vi "运维调试_总磷总氮.vi"() -> ()   [LabVIEW 2016, in "斯坦道总磷.lvlib"]
uses:
  <vilib>/Utility/miscctls.llb/LVStringsAndValuesArrayTypeDef_U16.ctl
  <vilib>/Utility/miscctls.llb/LVPointTypeDef.ctl
  <vilib>/Plasmionique/MB Master/MB_Master/MB_Master.lvclass
  <vilib>/Utility/config.llb/NI_LVConfig.lvlib
  <vilib>/ptbypt/NI_PtbyPt.lvlib
panel:
  in  "测试量程配置":T1
  in  "启动参数设置":bool
  out "固件版本号":string
  in  "定时设置":cluster{"启动":bool, "控制命令":T2, "测量参数":T3}(xcontrol)
  out "模块版本号":string
  out "温度2":sgl
  out "温度1":sgl
  out "ADC":sgl
  out "F3":sgl format="%#.6f"
  out "F2":sgl format="%#.6f"
  out "F1":sgl format="%#.6f"
  out "F0":sgl format="%#.6f"
  out "运行状态":T4 {"数据时间:" format="%<%y/%m/%d %H:%M:%S>T"; "仪器时间:" format="%<%y/%m/%d %H:%M:%S>T"}
  in  "单选按钮":enum32{"COD", "NH3N", "TN", "TP"}(radio)=enum."TN"
  in  "仪器参数":bool
  out "二级权限":bool
  out "一级权限":bool
  out "输入密码":u32
  out "布尔":bool
  in  "流程固件":bool
  in  "量程参数读取":T5
  in  "模块启用":bool
  in  "串口设置":bool
  in  "公式一键写入":bool
  in  "流程路径":path=path "data/流程.xml"
  in  "曲线模型":cluster{"X^2":dbl, "X":dbl, "B":dbl, "r^2":dbl}(xcontrol)
  out "字符串 2":string
  in  "质控参数设置":bool
  in  "数组":string[](array[string])
  in  "量程切换阈值写入":bool
  in  "量程切换阈值读取":bool
  in  "参数下拉列表":enum16{"COD", "氨氮", "总氮", "总磷"}(ring)
  in  "量程下拉列表":enum16{"低量程", "高量程"}(ring)
  in  "测量模式下拉列表":enum16{"水样测量", "零点核查", "跨度核查", "标样核查", "加标回收"}(ring)
  in  "公式":cluster{"X^2":dbl, "X":dbl, "b":dbl}
  in  "写公式":bool
  in  "读公式":bool
  in  "返回":bool
  in  "参数设置":bool
  out "集成报警信息":string
  in  "停止":bool
  in  "手动启动":bool
  in  "单步测试":bool
  out "多列列表框":i32(listbox)
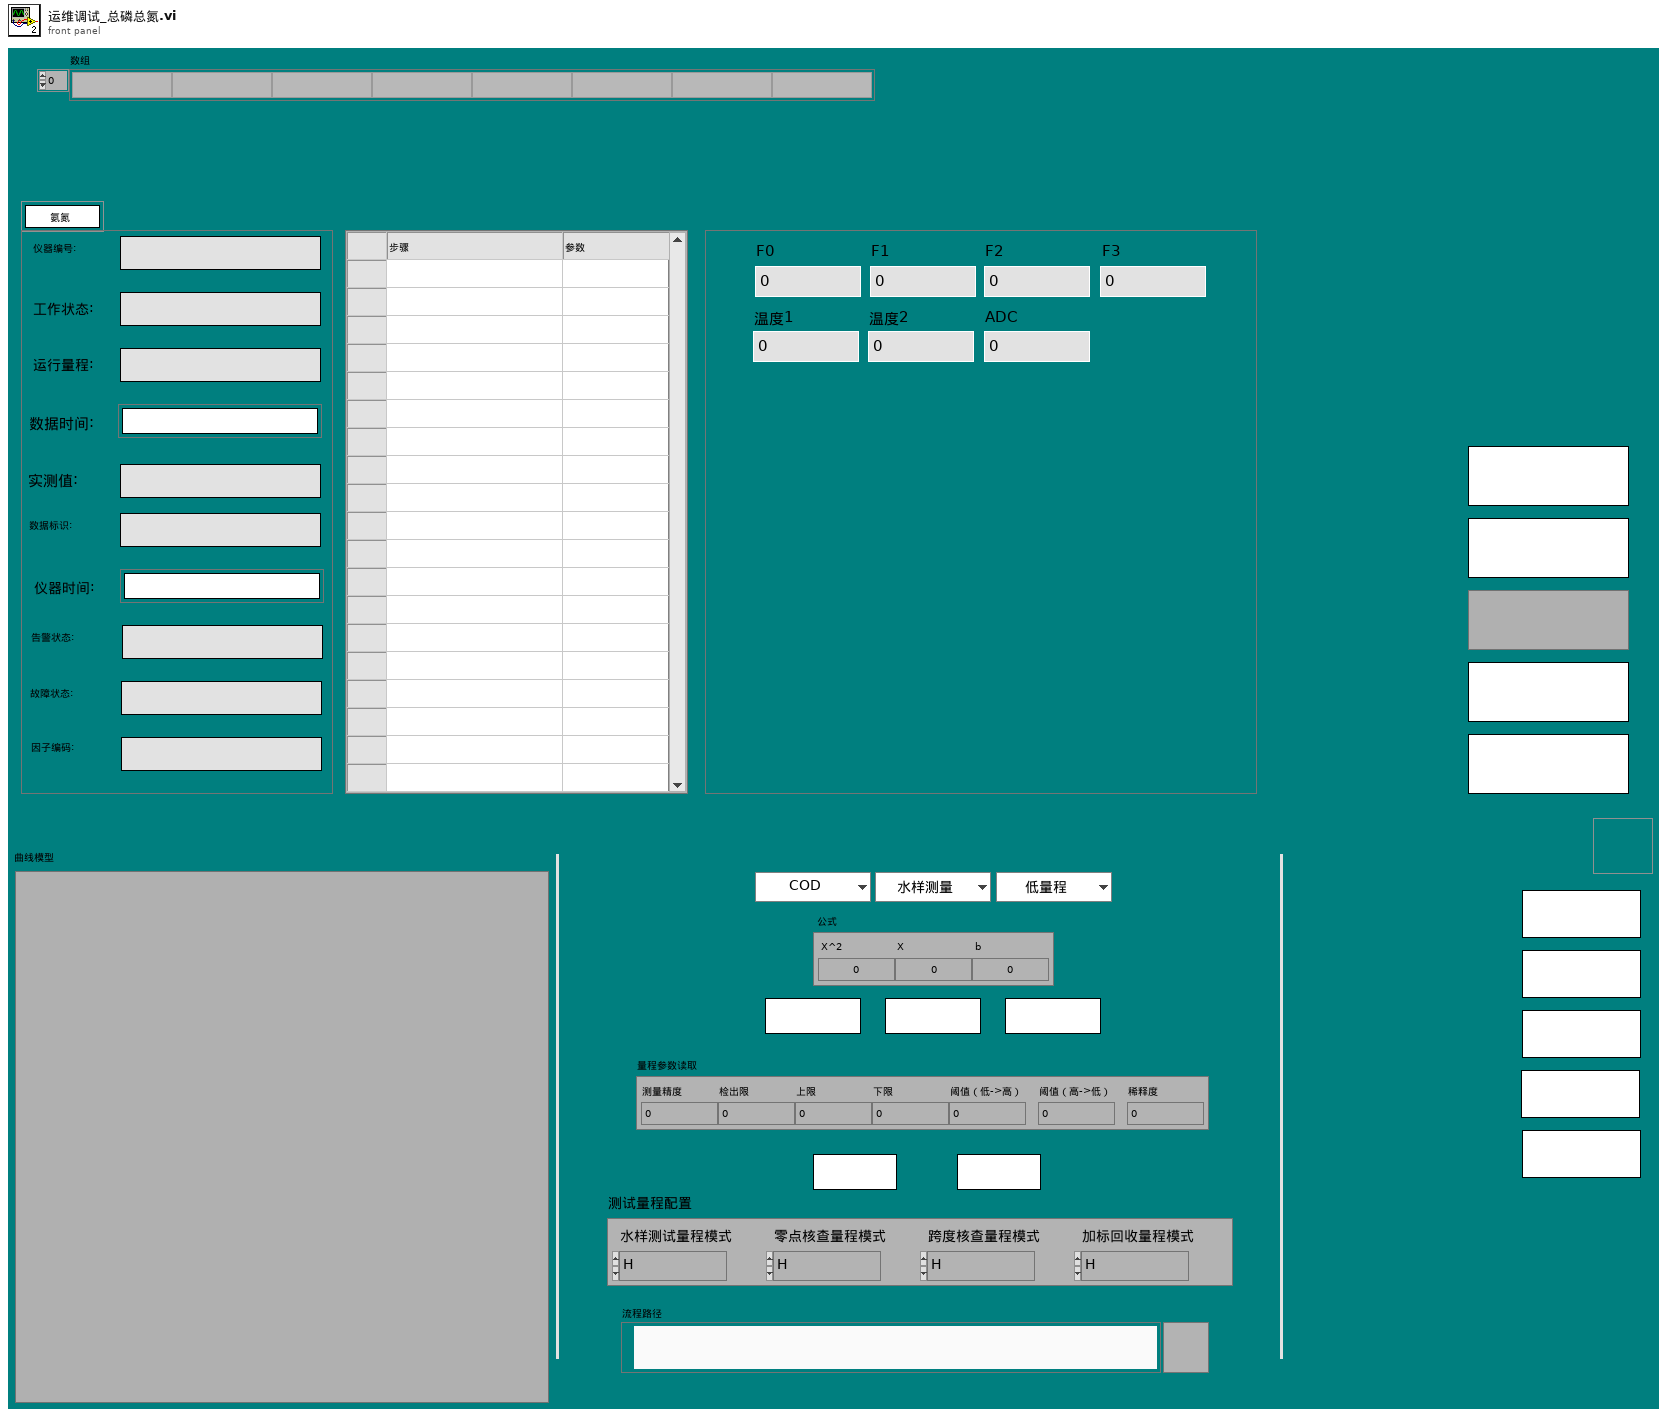
[diagram p1: front panel]
types:
  T1 = cluster{"水样测试量程模式":enum16{"H", "L", "AUTO"}, "空白核查量程模式":enum16{"H", "L", "AUTO"}, "跨度核查量程模式":enum16{"H", "L", "AUTO"}, "跨度核查量程模式 2":enum16{"H", "L", "AUTO"}}
  T2 = typedef "定时设置.xctl/国标控制命令.ctl" = enum16{"启动测量", "标样核查", "零点核查", "跨度核查", "空白测试", "平行样测试", "加标回收", "空白校准", "标样校准", "初始化（清洗）", "停止测试", "仪器重启", "校时", "模式设置", "测量间隔设置"}
  T3 = typedef "定时设置.xctl/测量参数.ctl" = u16
  T4 = cluster{"仪器编号:":string, "工作状态:":string, "运行量程: ":string, "数据时间:":timestamp, "实测值:":string, "数据标识: ":string, "仪器时间:":timestamp, "告警状态: ":string, "故障状态:  ":string, "因子编码:":string}
  T5 = cluster{"测量精度":dbl, "检出限":dbl, "上限":dbl, "下限":dbl, "阈值（低->高）":dbl, "阈值（高->低）":dbl, "稀释度":dbl}
  T6 = cluster{"时间源选择":enum16{"系统时间源", "仪器时间源"}, "外部时间源":timestamp}
  T7 = cluster{"系统时间":timestamp, "工作状态":enum16{"空闲", "水样测试", "标样核查", "零点核查", "跨度核查", "空白测试", "平行样测试", "加标回收", "空白校准", "标样校准", "初始化（清洗）"}, "测量模式":enum16{"待机", "连续模式", "周期模式", "定点模式", "受控模式", "手动模式"}, "告警代码":u16, "故障代码":u16, "日志代码":u16, "软件版本":u16, "F0":sgl, "F1":sgl, "F2":sgl, "F3":sgl, "T":sgl, "H":sgl, "id":u16, "flowid":u16, "量程":u16, "总磷控温温度1":sgl, "营养盐控温温度2":sgl, "ADC":sgl}
  T8 = enum32{"Bad", "Idle", "Run top level", "Running"}
  T9 = enum16{"空闲", "水样测试", "标样核查", "零点核查", "跨度核查", "空白测试", "平行样测试", "加标回收", "空白校准", "标样校准", "初始化（清洗）"}
  T10 = cluster{"水样测试量程模式":enum16{"H", "L", "AUTO"}, "空白核查量程模式":enum16{"H", "L", "AUTO"}, "跨度核查量程模式":enum16{"H", "L", "AUTO"}, "加标回收量程模式":enum16{"H", "L", "AUTO"}}
  T11 = typedef "LVStringsAndValuesArrayTypeDef_U16.ctl" = cluster{"String":string, "Value":u16}[]
  T12 = cluster{"COD":bool, "氨氮":bool, "总氮":bool, "总磷":bool}
  T13 = typedef "NI_LVConfig.lvlib/Config Data RefNum.ctl" = refnum<k1>
  T14 = cluster{"Major":u16, "Minor":u16, "Fix":u16, "Build":u16}
  T15 = cluster{i32, "测量模式下拉列表":enum16{"水样测量", "零点核查", "跨度核查", "标样核查", "加标回收"}, "量程下拉列表":enum16{"低量程", "高量程"}}
  T16 = typedef "LVPointTypeDef.ctl" = cluster{"Horizontal":i16, "Vertical":i16}
  T17 = cluster{"因子编码":u32, "单位":u16, "标样参考值":sgl, "水样数据时间":timestamp, "水样实测值":sgl, "水样数据标识":string, "标样数据时间":timestamp, "标样实测值":sgl, "标样数据标识":string, "空白数据时间":timestamp, "空白实测值":sgl, "空白数据标识":string, "零点核查数据时间":timestamp, "零点核查实测值":sgl, "零点核查数据标识":string, "跨度核查数据时间":timestamp, "跨度核查实测值":sgl, "跨度核查数据标识":string, "加标回收数据时间":timestamp, "加标回收实测值":sgl, "加标回收数据标识":string, "平行样数据时间":timestamp, "平行样实测值":sgl, "平行样数据标识":string, "F0":sgl, "F1":sgl, "F2":sgl, "F3":sgl, "F4":sgl, "F5":sgl, "F6":sgl, "F7":sgl, "温度":sgl, "湿度":sgl, "X值":sgl, "fidrange":u16}
  T18 = cluster{"时间标识":timestamp, "设备":string, "日志信息":string, "备注":string}
  T19 = cluster{"参数":string, "报警内容":string, "报警分析":string}
  T20 = cluster{"启动模式":enum16{"跨度核查", "水样测量", "空白核查", "标样核查", "加标回收"}, "启动参数":u16, "量程":enum16{"低量程", "高量程"}}
  T21 = cluster{"时间标识":timestamp, "设备":string, "日志信息":string, "流程参数":string}
  T22 = typedef "LVRowAndColumnUnsignedTypeDef.ctl" = cluster{"Row":u32, "Column":u32}
  T23 = cluster{"站号":u16, "量程切换":enum32{"H", "L", "AUTO"}, "控制命令":enum16{"启动测量", "标样核查", "零点核查", "跨度核查", "空白测试", "平行样测试", "加标回收", "空白校准", "标样校准", "初始化（清洗）", "停止测试", "仪器重启", "校时", "模式设置", "测量间隔设置"}, "模式设置":enum16{"待机", "连续模式", "周期模式", "定点模式", "受控模式", "手动模式"}, "测量间隔":u16}
  T24 = cluster{"参数下拉列表":enum16{"COD", "氨氮", "总氮", "总磷"}, "测量模式下拉列表":enum16{"水样测量", "零点核查", "跨度核查", "标样核查", "加标回收"}, "量程下拉列表":enum16{"低量程", "高量程"}}
  T25 = cluster{"被复制模型":cluster{"参数":u8, "测量模式":u8, "量程":u8}, "被覆盖模型":cluster{"参数":u8, "测量模式":u8, "量程":u8}[]}
  T26 = cluster{"总磷跨度值":dbl, "总磷零点标准液浓度":dbl, "总磷跨度标准液浓度":dbl, "总磷标准液标准浓度":dbl, "总氮跨度值":dbl, "总氮零点标准液浓度":dbl, "总氮跨度标准液浓度":dbl, "总氮标准液标准浓度":dbl, "COD跨度值":dbl, "COD零点标准液浓度":dbl, "COD跨度标准液浓度":dbl, "COD标准液标准浓度":dbl, "氨氮跨度值":dbl, "氨氮零点标准液浓度":dbl, "氨氮跨度标准液浓度":dbl, "氨氮标准液标准浓度":dbl}
  T27 = cluster{"测量量程":dbl, "测量精度":dbl, "测量间隔":dbl, "消解温度":dbl, "消解时长":dbl, "空白校准时间":timestamp, "曲线截距":dbl, "曲线斜率":dbl, "测量检出限":dbl, "测量信号值":dbl, "线性相关系数":dbl, "二次多项式系数":dbl, "标样校准时间":timestamp, "稀释倍数":dbl, "三项式系数":dbl, "空白标定系数":dbl, "量程系数":dbl, "F0/ORPA":dbl, "F1/ORPB":dbl, "F2/ORPK":dbl, "F3":dbl, "F4":dbl, "F5":dbl, "F6":dbl, "F7":dbl, "X0/滴定数":dbl, "量程":dbl}
  T28 = cluster{"COD仪器参数":cluster{"测量量程":dbl, "测量精度":dbl, "测量间隔":dbl, "消解温度":dbl, "消解时长":dbl, "空白校准时间":timestamp, "曲线截距":dbl, "曲线斜率":dbl, "测量检出限":dbl, "测量信号值":dbl, "线性相关系数":dbl, "二次多项式系数":dbl, "标样校准时间":timestamp, "稀释倍数":dbl, "三项式系数":dbl, "空白标定系数":dbl, "量程系数":dbl, "F0/ORPA":dbl, "F1/ORPB":dbl, "F2/ORPK":dbl, "F3":dbl, "F4":dbl, "F5":dbl, "F6":dbl, "F7":dbl, "X0/滴定数":dbl, "量程":dbl}, "氨氮仪器参数":cluster{"测量量程":dbl, "测量精度":dbl, "测量间隔":dbl, "消解温度":dbl, "消解时长":dbl, "空白校准时间":timestamp, "曲线截距":dbl, "曲线斜率":dbl, "测量检出限":dbl, "测量信号值":dbl, "线性相关系数":dbl, "二次多项式系数":dbl, "标样校准时间":timestamp, "稀释倍数":dbl, "三项式系数":dbl, "空白标定系数":dbl, "量程系数":dbl, "F0/ORPA":dbl, "F1/ORPB":dbl, "F2/ORPK":dbl, "F3":dbl, "F4":dbl, "F5":dbl, "F6":dbl, "F7":dbl, "X0/滴定数":dbl, "量程":dbl}, "总氮仪器参数":cluster{"测量量程":dbl, "测量精度":dbl, "测量间隔":dbl, "消解温度":dbl, "消解时长":dbl, "空白校准时间":timestamp, "曲线截距":dbl, "曲线斜率":dbl, "测量检出限":dbl, "测量信号值":dbl, "线性相关系数":dbl, "二次多项式系数":dbl, "标样校准时间":timestamp, "稀释倍数":dbl, "三项式系数":dbl, "空白标定系数":dbl, "量程系数":dbl, "F0/ORPA":dbl, "F1/ORPB":dbl, "F2/ORPK":dbl, "F3":dbl, "F4":dbl, "F5":dbl, "F6":dbl, "F7":dbl, "X0/滴定数":dbl, "量程":dbl}, "总磷仪器参数":cluster{"测量量程":dbl, "测量精度":dbl, "测量间隔":dbl, "消解温度":dbl, "消解时长":dbl, "空白校准时间":timestamp, "曲线截距":dbl, "曲线斜率":dbl, "测量检出限":dbl, "测量信号值":dbl, "线性相关系数":dbl, "二次多项式系数":dbl, "标样校准时间":timestamp, "稀释倍数":dbl, "三项式系数":dbl, "空白标定系数":dbl, "量程系数":dbl, "F0/ORPA":dbl, "F1/ORPB":dbl, "F2/ORPK":dbl, "F3":dbl, "F4":dbl, "F5":dbl, "F6":dbl, "F7":dbl, "X0/滴定数":dbl, "量程":dbl}}
  T29 = cluster{"测量精度":u16, "检出限":dbl, "上限":dbl, "下限":dbl, "阈值（低->高）":dbl, "阈值（高->低）":dbl, "稀释度":dbl}
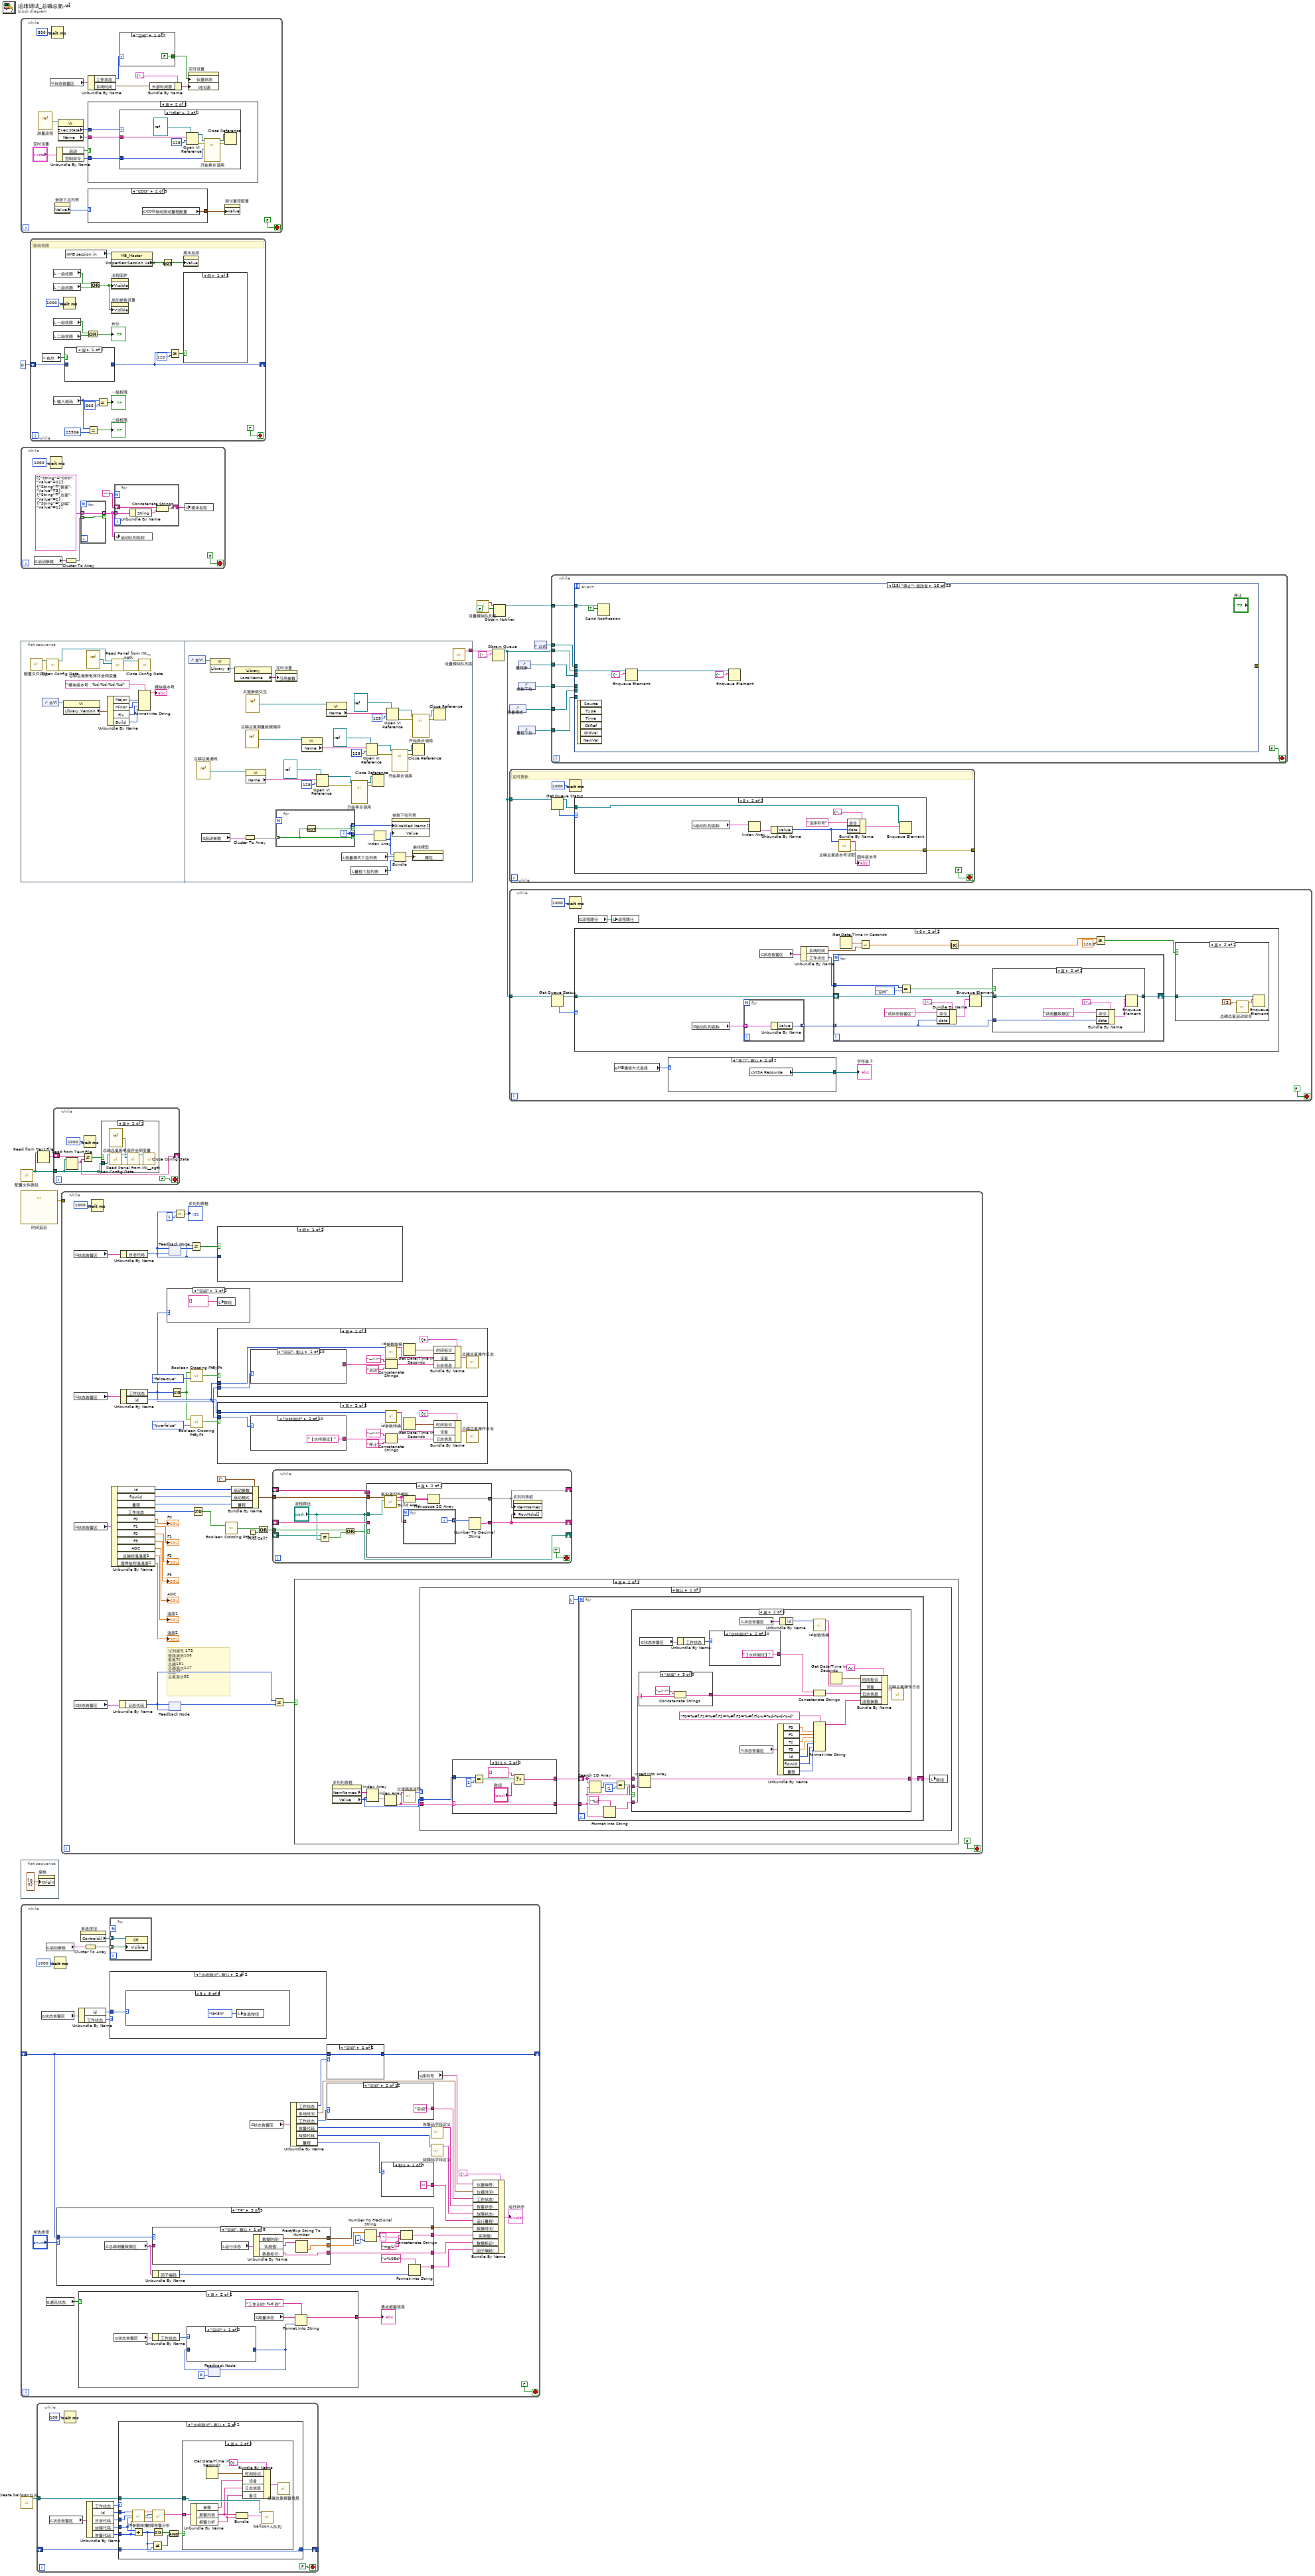
[diagram p0: block diagram]
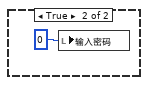
[diagram p5: hidden frame]
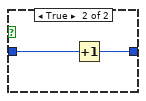
[diagram p6: hidden frame]
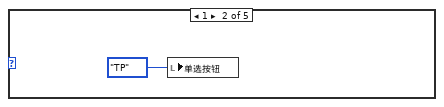
[diagram p11: hidden frame]
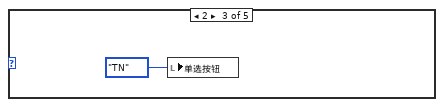
[diagram p12: hidden frame]
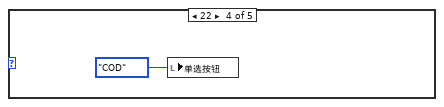
[diagram p13: hidden frame]
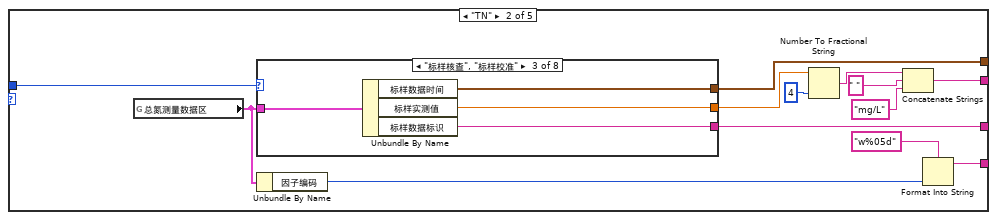
[diagram p15: hidden frame]
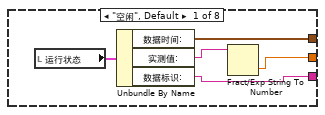
[diagram p16: hidden frame]
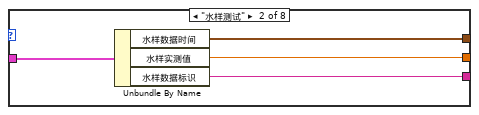
[diagram p17: hidden frame]
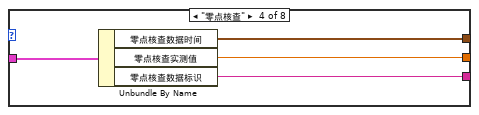
[diagram p18: hidden frame]
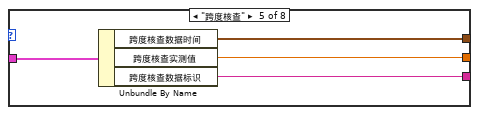
[diagram p19: hidden frame]
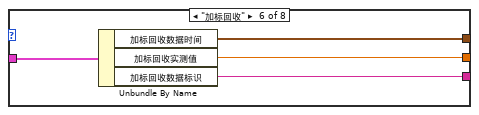
[diagram p20: hidden frame]
diagram:
  n1 = while {
    stop <- FALSE stop-if-true
    n2 = vi-ref "测量流程.vi"() -> (w30:refnum<vi>)
    n3 = global read "VAR总磷总氮全局变量.vi" "状态告警区"() -> (w27:T7)
    n4 = Wait (ms)(milliseconds to wait=u32 500 ("等待时间（毫秒）")) -> ()  [unwired: 1 out]
    n5 = property on="参数下拉列表" class="Enum (严格)"() -> ("Value"=w19:enum16{"COD", "氨氮", "总氮", "总磷"})  [unwired: 2 in, 2 out]
    n6 = Unbundle By Name("定时设置") -> ("启动"=w24:bool, "控制命令"=w23:T2)
    n7 = property class="VI"(reference=w30) -> ("Exec.State"=w29:T8, "Name"=w28:string)  [unwired: 1 in, 2 out]
    n8 = Unbundle By Name(w27) -> ("工作状态"=w26:T9, "系统时间"=w21:timestamp)
    n9 = case shown="真" w24 {
      tunnel: w28 -> [_ w41]
      tunnel: w23 -> [_ w40]
      tunnel: w29 -> [_ w39]
      frame False {
      }
      frame True {
        n10 = case shown="\"Idle\"" w39 {
          tunnel: w41 -> [_ w45]
          tunnel: w40 -> [_ w42]
          frame "Bad", Default {
          }
          frame "Idle" {
            n11 = Open VI Reference(type specifier VI Refnum (for type only)=refnum<vi> refnum, vi path=w45, options=128 ("选项")) -> (vi reference=w46:refnum<vi>, error out=w47:errorcluster)  [unwired: 3 in]
            n12 = call-by-ref "开始异步调用"(reference=w46, error in=w47, "控制命令"=w42) -> (reference out=w48:refnum<vi>, error out=w49:errorcluster)  [unwired: 11 in]
            n13 = Close Reference(reference=w48, error in (no error)=w49) -> ()  [unwired: 1 out]
          }
        }
      }
    }
    n14 = case shown="\"COD\"" w19 {
      tunnel: [_ w33 w34 w35 w36] -> w18
      frame Default {
      }
      frame "COD" {
        n15 = global read "总磷总氮断电保存全局变量.vi" "COD自动测试量程配置"() -> (w33:T10)
      }
      frame "氨氮" {
        n16 = global read "总磷总氮断电保存全局变量.vi" "氨氮自动测试量程配置"() -> (w34:T10)
      }
      frame "总氮" {
        n17 = global read "总磷总氮断电保存全局变量.vi" "总氮自动测试量程配置"() -> (w35:T10)
      }
      frame "总磷" {
        n18 = global read "总磷总氮断电保存全局变量.vi" "总磷自动测试量程配置"() -> (w36:T10)
      }
    }
    n19 = case shown="\"空闲\"" w26 {
      tunnel: [FALSE TRUE] -> w17
      frame "空闲" {
      }
      frame "水样测试", Default {
      }
    }
    n20 = Bundle By Name(cluster=T6 {"时间源选择"=enum."仪器时间源", "外部时间源"=timestamp(0 s since 1904-01-01)} ("时间源"), "外部时间源"=w21) -> (w20:T6)
    n21 = property on="定时设置" class="定时设置 (严格)"("仪器状态"=w17, "时间源"=w20) -> ()  [unwired: 2 in, 2 out]
    n22 = property on="测试量程配置" class="Clust (严格)"("Value"=w18) -> ()  [unwired: 2 in, 2 out]
  }
  n23 = while {
    stop <- FALSE stop-if-true
    n24 = global read "总磷总氮断电保存全局变量.vi" "启动参数"() -> (w55:T12)
    n25 = Wait (ms)(milliseconds to wait=u32 1000 ("等待时间（毫秒）")) -> ()  [unwired: 1 out]
    n26 = Cluster To Array(cluster=w55) -> (array=w54:bool[])
    n27 = for {
      tunnel: w54 -> [w63] mode=indexing
      tunnel: T11 [{"String"="COD", "Value"=22}, {"String"="氨氮", "Value"=3}, {"String"="总氮", "Value"=2}, {"String"="总磷", "Value"=1}] ("字符串与值[]") -> [w62] mode=indexing
      tunnel: [w62] -> w52 mode=indexing if=w63
    }
    n28 = for {
      tunnel: w52 -> [w61] mode=indexing
      shift-right: [w60] -> w50
      shift-left: "" -> [w58]
      n29 = Unbundle By Name(w61) -> ("String"=w59:string)
      n30 = Concatenate Strings(w58, w59) -> (w60:string)
    }
    n31 = global write "VAR总磷总氮全局变量.vi" "启动队列名称"(w52) -> ()
    n32 = global write "VAR总磷总氮全局变量.vi" "模块名称"(w50) -> ()
  }
  n33 = flat-sequence {
    tunnel: [w78] -> w6
    frame #0 {
      n34 = call "配置文件路径.vi"() -> ("appended path"=w72:path)  [unwired: 11 in]
      n35 = control-ref of="本VI"() -> (w71:refnum<vi>)
      n36 = call <vilib>:"Open Config Data.vi"("configuration file path"=w72) -> ("error out"=w76:errorcluster, "refnum"=w73:T13)  [unwired: 8 in, 1 out]
      n37 = property class="VI"(reference=w71) -> ("Library.Version"=w70:T14)  [unwired: 1 in, 2 out]
      n38 = vi-ref "总磷总氮断电保存全局变量.vi"() -> (w74:refnum<vi>)
      n39 = Unbundle By Name(w70) -> ("Major"=w68:u16, "Minor"=w67:u16, "Fix"=w66:u16, "Build"=w65:u16)
      n40 = call <userlib>:"Read Panel from INI__ogtk.vi"("error in (no error)"=w76, "VI ref"=w74, "refnum"=w73) -> ("error out"=w77:errorcluster, "refnum out"=w75:T13)  [unwired: 7 in]
      n41 = call <vilib>:"Close Config Data.vi"("error in (no error)"=w77, "refnum"=w75) -> ()  [unwired: 8 in, 2 out]
      n42 = Format Into String(format string="模块版本号：%d.%d.%d.%d" ("格式字符串"), w68, w67, w66, w65) -> (resulting string=→"模块版本号":string)  [unwired: 2 in, 1 out]
    }
    frame #1 {
      n43 = control-ref of="本VI"() -> (w80:refnum<vi>)
      n44 = vi-ref "总磷总氮通讯.vi"() -> (w98:refnum<vi>)
      n45 = global read "总磷总氮断电保存全局变量.vi" "启动参数"() -> (w86:T12)
      n46 = property class="VI"(reference=w80) -> ("Library"=w81:refnum<vi>)  [unwired: 1 in, 2 out]
      n47 = property class="Library"(reference=w81) -> ("LocalName"=w82:string)  [unwired: 1 in, 2 out]
      n48 = Cluster To Array(cluster=w86) -> (array=w87:bool[])
      n49 = vi-ref "总磷总氮测量数据储存.vi"() -> (w106:refnum<vi>)
      n50 = vi-ref "关键参数交互.vi"() -> (w97:refnum<vi>)
      n51 = property class="VI"(reference=w98) -> ("Name"=w99:string)  [unwired: 1 in, 2 out]
      n52 = property on="定时设置" class="定时设置 (严格)"("引用参数"=w82) -> ()  [unwired: 2 in, 2 out]
      n53 = for {
        tunnel: w87 -> [w114] mode=indexing
        tunnel: [w115] -> w89 mode=indexing if=w116
        tunnel: [w115] -> w88 mode=indexing if=w114
        i -> [w115]
        n54 = Not(x=w114) -> (.not. x?=w116:bool)
      }
      n55 = property class="VI"(reference=w106) -> ("Name"=w113:string)  [unwired: 1 in, 2 out]
      n56 = Open VI Reference(type specifier VI Refnum (for type only)=refnum<vi> refnum, vi path=w99, options=128 ("选项")) -> (vi reference=w101:refnum<vi>, error out=w103:errorcluster)  [unwired: 3 in]
      n57 = property class="VI"(reference=w97) -> ("Name"=w91:string)  [unwired: 1 in, 2 out]
      n58 = local read "测量模式下拉列表"() -> (w84:enum16{"水样测量", "零点核查", "跨度核查", "标样核查", "加标回收"})
      n59 = local read "量程下拉列表"() -> (w83:enum16{"低量程", "高量程"})
      n60 = call-by-ref "开始异步调用"(reference=w101, error in=w103) -> (reference out=w105:refnum<vi>, error out=w104:errorcluster)  [unwired: 12 in]
      n61 = Open VI Reference(type specifier VI Refnum (for type only)=refnum<vi> refnum, vi path=w113, options=128 ("选项")) -> (vi reference=w111:refnum<vi>, error out=w109:errorcluster)  [unwired: 3 in]
      n62 = Close Reference(reference=w105, error in (no error)=w104) -> ()  [unwired: 1 out]
      n63 = Index Array(array=w88) -> (element=w79:i32)  [unwired: 1 in]
      n64 = Open VI Reference(type specifier VI Refnum (for type only)=refnum<vi> refnum, vi path=w91, options=128 ("选项")) -> (vi reference=w93:refnum<vi>, error out=w94:errorcluster)  [unwired: 3 in]
      n65 = call-by-ref "开始异步调用"(reference=w111, error in=w109) -> (reference out=w107:refnum<vi>, error out=w108:errorcluster)  [unwired: 12 in]
      n66 = property on="参数下拉列表" class="Enum (严格)"("Disabled Items []"=w89, "Value"=w79) -> ()  [unwired: 2 in, 2 out]
      n67 = Bundle(w79, "测量模式下拉列表"=w84, "量程下拉列表"=w83) -> (w85:T15)  [unwired: 1 in]
      n68 = call-by-ref "开始异步调用"(reference=w93, error in=w94) -> (reference out=w96:refnum<vi>, error out=w95:errorcluster)  [unwired: 12 in]
      n69 = Close Reference(reference=w107, error in (no error)=w108) -> ()  [unwired: 1 out]
      n70 = property on="曲线模型" class="曲线模型 (严格)"("属性"=w85) -> ()  [unwired: 2 in, 2 out]
      n71 = Close Reference(reference=w96, error in (no error)=w95) -> ()  [unwired: 1 out]
      n72 = call "设置模块队列名.vi"() -> ("Msg"=w78:string)  [unwired: 5 in]
    }
  }
  n73 = call "配置文件路径.vi"() -> ("appended path"=w4:path)  [unwired: 11 in]
  n74 = call "时间延迟"() -> ("error out"=w11:errorcluster)  [unwired: 11 in]
  n75 = flat-sequence {
    frame #0 {
      n76 = property on="窗格" class="Pane"("Origin"=T16 {"Horizontal"=0, "Vertical"=0} ("原点")) -> ()  [unwired: 2 in, 2 out]
    }
  }
  n77 = while {
    shift-right: [w119] -> _
    shift-left: _ -> [w118]
    stop <- FALSE stop-if-true
    n78 = global read "VAR总磷总氮全局变量.vi" "状态告警区"() -> (w130:T7)
    n79 = global read "总磷总氮断电保存全局变量.vi" "启动参数"() -> (w122:T12)
    n80 = global read "VAR总磷总氮全局变量.vi" "通讯状态"() -> (w146:bool)
    n81 = Wait (ms)(milliseconds to wait=u32 1000 ("等待时间（毫秒）")) -> ()  [unwired: 1 out]
    n82 = case shown="\"TP\"" "单选按钮" {
      tunnel: w118 -> [_ w162 w208 w254 w300]
      tunnel: [_ w161 w207 w252 w298] -> w134
      tunnel: [_ w160 w210 w256 w302] -> w133
      tunnel: [_ w159 w205 w250 w296] -> w132
      tunnel: [_ w158 w209 w255 w301] -> w131
      frame Default {
      }
      frame "TN" {
        n83 = global read "VAR总磷总氮全局变量.vi" "总氮测量数据区"() -> (w163:T17)
        n84 = case shown="\"标样核查\", \"标样校准\"" w162 {
          tunnel: [w173 w179 w183 w187 w191 w195 w199 w203] -> w161
          tunnel: [w171 w178 w182 w186 w189 w194 w198 w202] -> w165
          tunnel: [w174 w177 w181 w185 w188 w193 w197 w201] -> w159
          tunnel: w163 -> [_ w176 w180 w184 w190 w192 w196 w200]
          frame "空闲", Default {
            n85 = local read "运行状态"() -> (w175:T4)
            n86 = Unbundle By Name(w175) -> ("数据时间:"=w173:timestamp, "实测值:"=w172:string, "数据标识:"=w174:string)
            n87 = Fract/Exp String To Number(string=w172) -> (number=w171:dbl)  [unwired: 3 in, 1 out]
          }
          frame "水样测试" {
            n88 = Unbundle By Name(w176) -> ("水样数据时间"=w179:timestamp, "水样实测值"=w178:sgl, "水样数据标识"=w177:string)
          }
          frame "标样核查", "标样校准" {
            n89 = Unbundle By Name(w180) -> ("标样数据时间"=w183:timestamp, "标样实测值"=w182:sgl, "标样数据标识"=w181:string)
          }
          frame "零点核查" {
            n90 = Unbundle By Name(w184) -> ("零点核查数据时间"=w187:timestamp, "零点核查实测值"=w186:sgl, "零点核查数据标识"=w185:string)
          }
          frame "跨度核查" {
            n91 = Unbundle By Name(w190) -> ("跨度核查数据时间"=w191:timestamp, "跨度核查实测值"=w189:sgl, "跨度核查数据标识"=w188:string)
          }
          frame "加标回收" {
            n92 = Unbundle By Name(w192) -> ("加标回收数据时间"=w195:timestamp, "加标回收实测值"=w194:sgl, "加标回收数据标识"=w193:string)
          }
          frame "空白测试", "空白校准" {
            n93 = Unbundle By Name(w196) -> ("空白数据时间"=w199:timestamp, "空白实测值"=w198:sgl, "空白数据标识"=w197:string)
          }
          frame "平行样测试" {
            n94 = Unbundle By Name(w200) -> ("平行样数据时间"=w203:timestamp, "平行样实测值"=w202:sgl, "平行样数据标识"=w201:string)
          }
        }
        n95 = Unbundle By Name(w163) -> ("因子编码"=w169:u32)
        n96 = Number To Fractional String(number=w165, precision (6)=i16 4 ("精度(6)")) -> (F-format string=w167:string)  [unwired: 2 in]
        n97 = Concatenate Strings(w167, " " ("字符串"), "mg/L" ("字符串")) -> (w160:string)
        n98 = Format Into String(format string="w%05d" ("格式字符串"), w169) -> (resulting string=w158:string)  [unwired: 2 in, 1 out]
      }
      frame "TP" {
        n99 = global read "VAR总磷总氮全局变量.vi" "总磷测量数据区"() -> (w204:T17)
        n100 = case shown="\"空闲\", 默认" w208 {
          tunnel: [w219 w225 w229 w233 w237 w241 w245 w249] -> w207
          tunnel: [w217 w224 w228 w232 w235 w240 w244 w248] -> w206
          tunnel: [w220 w223 w227 w231 w234 w239 w243 w247] -> w205
          tunnel: w204 -> [_ w222 w226 w230 w236 w238 w242 w246]
          frame "空闲", Default {
            n101 = local read "运行状态"() -> (w221:T4)
            n102 = Unbundle By Name(w221) -> ("数据时间:"=w219:timestamp, "实测值:"=w218:string, "数据标识:"=w220:string)
            n103 = Fract/Exp String To Number(string=w218) -> (number=w217:dbl)  [unwired: 3 in, 1 out]
          }
          frame "水样测试" {
            n104 = Unbundle By Name(w222) -> ("水样数据时间"=w225:timestamp, "水样实测值"=w224:sgl, "水样数据标识"=w223:string)
          }
          frame "标样核查" {
            n105 = Unbundle By Name(w226) -> ("标样数据时间"=w229:timestamp, "标样实测值"=w228:sgl, "标样数据标识"=w227:string)
          }
          frame "零点核查" {
            n106 = Unbundle By Name(w230) -> ("零点核查数据时间"=w233:timestamp, "零点核查实测值"=w232:sgl, "零点核查数据标识"=w231:string)
          }
          frame "跨度核查" {
            n107 = Unbundle By Name(w236) -> ("跨度核查数据时间"=w237:timestamp, "跨度核查实测值"=w235:sgl, "跨度核查数据标识"=w234:string)
          }
          frame "加标回收" {
            n108 = Unbundle By Name(w238) -> ("加标回收数据时间"=w241:timestamp, "加标回收实测值"=w240:sgl, "加标回收数据标识"=w239:string)
          }
          frame "空白测试" {
            n109 = Unbundle By Name(w242) -> ("空白数据时间"=w245:timestamp, "空白实测值"=w244:sgl, "空白数据标识"=w243:string)
          }
          frame "平行样测试" {
            n110 = Unbundle By Name(w246) -> ("平行样数据时间"=w249:timestamp, "平行样实测值"=w248:sgl, "平行样数据标识"=w247:string)
          }
        }
        n111 = Unbundle By Name(w204) -> ("因子编码"=w215:u32)
        n112 = Number To Fractional String(number=w206, precision (6)=i16 4 ("精度(6)")) -> (F-format string=w213:string)  [unwired: 2 in]
        n113 = Concatenate Strings(w213, " " ("字符串"), "mg/L" ("字符串")) -> (w210:string)
        n114 = Format Into String(format string="w%05d" ("格式字符串"), w215) -> (resulting string=w209:string)  [unwired: 2 in, 1 out]
      }
      frame "NH3N" {
        n115 = global read "VAR总磷总氮全局变量.vi" "氨氮测量数据区"() -> (w253:T17)
        n116 = case shown="\"空闲\", 默认" w254 {
          tunnel: [w265 w271 w275 w279 w283 w287 w291 w295] -> w252
          tunnel: [w263 w270 w274 w278 w281 w286 w290 w294] -> w251
          tunnel: [w266 w269 w273 w277 w280 w285 w289 w293] -> w250
          tunnel: w253 -> [_ w268 w272 w276 w282 w284 w288 w292]
          frame "空闲", Default {
            n117 = local read "运行状态"() -> (w267:T4)
            n118 = Unbundle By Name(w267) -> ("数据时间:"=w265:timestamp, "实测值:"=w264:string, "数据标识:"=w266:string)
            n119 = Fract/Exp String To Number(string=w264) -> (number=w263:dbl)  [unwired: 3 in, 1 out]
          }
          frame "水样测试" {
            n120 = Unbundle By Name(w268) -> ("水样数据时间"=w271:timestamp, "水样实测值"=w270:sgl, "水样数据标识"=w269:string)
          }
          frame "标样核查" {
            n121 = Unbundle By Name(w272) -> ("标样数据时间"=w275:timestamp, "标样实测值"=w274:sgl, "标样数据标识"=w273:string)
          }
          frame "零点核查" {
            n122 = Unbundle By Name(w276) -> ("零点核查数据时间"=w279:timestamp, "零点核查实测值"=w278:sgl, "零点核查数据标识"=w277:string)
          }
          frame "跨度核查" {
            n123 = Unbundle By Name(w282) -> ("跨度核查数据时间"=w283:timestamp, "跨度核查实测值"=w281:sgl, "跨度核查数据标识"=w280:string)
          }
          frame "加标回收" {
            n124 = Unbundle By Name(w284) -> ("加标回收数据时间"=w287:timestamp, "加标回收实测值"=w286:sgl, "加标回收数据标识"=w285:string)
          }
          frame "空白测试" {
            n125 = Unbundle By Name(w288) -> ("空白数据时间"=w291:timestamp, "空白实测值"=w290:sgl, "空白数据标识"=w289:string)
          }
          frame "平行样测试" {
            n126 = Unbundle By Name(w292) -> ("平行样数据时间"=w295:timestamp, "平行样实测值"=w294:sgl, "平行样数据标识"=w293:string)
          }
        }
        n127 = Unbundle By Name(w253) -> ("因子编码"=w261:u32)
        n128 = Number To Fractional String(number=w251, precision (6)=i16 4 ("精度(6)")) -> (F-format string=w259:string)  [unwired: 2 in]
        n129 = Concatenate Strings(w259, " " ("字符串"), "mg/L" ("字符串")) -> (w256:string)
        n130 = Format Into String(format string="w%05d" ("格式字符串"), w261) -> (resulting string=w255:string)  [unwired: 2 in, 1 out]
      }
      frame "COD" {
        n131 = global read "VAR总磷总氮全局变量.vi" "COD测量数据区"() -> (w299:T17)
        n132 = case shown="\"空闲\", 默认" w300 {
          tunnel: [w311 w317 w321 w325 w329 w333 w337 w341] -> w298
          tunnel: [w309 w316 w320 w324 w327 w332 w336 w340] -> w297
          tunnel: [w312 w315 w319 w323 w326 w331 w335 w339] -> w296
          tunnel: w299 -> [_ w314 w318 w322 w328 w330 w334 w338]
          frame "空闲", Default {
            n133 = local read "运行状态"() -> (w313:T4)
            n134 = Unbundle By Name(w313) -> ("数据时间:"=w311:timestamp, "实测值:"=w310:string, "数据标识:"=w312:string)
            n135 = Fract/Exp String To Number(string=w310) -> (number=w309:dbl)  [unwired: 3 in, 1 out]
          }
          frame "水样测试" {
            n136 = Unbundle By Name(w314) -> ("水样数据时间"=w317:timestamp, "水样实测值"=w316:sgl, "水样数据标识"=w315:string)
          }
          frame "标样核查" {
            n137 = Unbundle By Name(w318) -> ("标样数据时间"=w321:timestamp, "标样实测值"=w320:sgl, "标样数据标识"=w319:string)
          }
          frame "零点核查" {
            n138 = Unbundle By Name(w322) -> ("零点核查数据时间"=w325:timestamp, "零点核查实测值"=w324:sgl, "零点核查数据标识"=w323:string)
          }
          frame "跨度核查" {
            n139 = Unbundle By Name(w328) -> ("跨度核查数据时间"=w329:timestamp, "跨度核查实测值"=w327:sgl, "跨度核查数据标识"=w326:string)
          }
          frame "加标回收" {
            n140 = Unbundle By Name(w330) -> ("加标回收数据时间"=w333:timestamp, "加标回收实测值"=w332:sgl, "加标回收数据标识"=w331:string)
          }
          frame "空白测试" {
            n141 = Unbundle By Name(w334) -> ("空白数据时间"=w337:timestamp, "空白实测值"=w336:sgl, "空白数据标识"=w335:string)
          }
          frame "平行样测试" {
            n142 = Unbundle By Name(w338) -> ("平行样数据时间"=w341:timestamp, "平行样实测值"=w340:sgl, "平行样数据标识"=w339:string)
          }
        }
        n143 = Unbundle By Name(w299) -> ("因子编码"=w307:u32)
        n144 = Number To Fractional String(number=w297, precision (6)=i16 4 ("精度(6)")) -> (F-format string=w305:string)  [unwired: 2 in]
        n145 = Concatenate Strings(w305, " " ("字符串"), "mg/L" ("字符串")) -> (w302:string)
        n146 = Format Into String(format string="w%05d" ("格式字符串"), w307) -> (resulting string=w301:string)  [unwired: 2 in, 1 out]
      }
    }
    n147 = Unbundle By Name(w130) -> ("id"=w129:u16, "工作状态"=w124:T9)
    n148 = case shown="真" w146 {
      tunnel: ["通讯异常" ("集成报警信息") w362] -> w145
      frame False {
      }
      frame True {
        n149 = global read "VAR总磷总氮全局变量.vi" "状态告警区"() -> (w368:T7)
        n150 = Unbundle By Name(w368) -> ("工作状态"=w367:T9)
        n151 = feedback #1(0) -> (w365:i32)
        n152 = case shown="\"空闲\"" w367 {
          tunnel: w365 -> [_ w370]
          tunnel: [_ w369] -> w363
          frame "空闲" {
          }
          frame Default {
            n153 = Increment(x=w370) -> (x+1=w369:i32)
          }
        }
        n154 = feedback-in #1(w363) -> ()
        n155 = global read "VAR总磷总氮全局变量.vi" "测量状态"() -> (w361:string)
        n156 = Format Into String(format string="工作计时: %d 秒" ("格式字符串"), initial string=w361, w363) -> (resulting string=w362:string)  [unwired: 1 in, 1 out]
      }
    }
    "集成报警信息" <- w145
    n157 = property on="单选按钮" class="RadioBtnsControl (严格)"() -> ("Controls[]"=w123:refnum<vi>[])  [unwired: 2 in, 2 out]
    n158 = Cluster To Array(cluster=w122) -> (array=w121:bool[])
    n159 = for {
      tunnel: w123 -> [w152] mode=indexing
      tunnel: w121 -> [w151] mode=indexing
      n160 = property class="Ctl"(reference=w152, "Visible"=w151) -> ()  [unwired: 1 in, 2 out]
    }
    n161 = case shown="\"水样测试\", 默认" w124 {
      tunnel: w129 -> [_ w153]
      frame "空闲" {
      }
      frame "水样测试", Default {
        n162 = case shown="3" w153 {
          frame 0, Default {
          }
          frame 1 {
            n163 = local write "单选按钮"(enum32{"COD", "NH3N", "TN", "TP"}."TP" ("单选按钮")) -> ()
          }
          frame 2 {
            n164 = local write "单选按钮"(enum32{"COD", "NH3N", "TN", "TP"}."TN" ("单选按钮")) -> ()
          }
          frame 22 {
            n165 = local write "单选按钮"(enum32{"COD", "NH3N", "TN", "TP"}."COD" ("单选按钮")) -> ()
          }
          frame 3 {
            n166 = local write "单选按钮"(enum32{"COD", "NH3N", "TN", "TP"}."NH3N" ("单选按钮")) -> ()
          }
        }
      }
    }
    n167 = global read "VAR总磷总氮全局变量.vi" "状态告警区"() -> (w144:T7)
    n168 = Unbundle By Name(w144) -> ("工作状态"=w120:T9, "系统时间"=w140:timestamp, "工作状态"=w139:T9, "告警代码"=w128:u16, "故障代码"=w126:u16, "量程"=w137:u16)
    n169 = case shown="\"空闲\"" w120 {
      selector: w120 -> [_ w150]
      tunnel: [w149 w150] -> w119
      tunnel: w118 -> [w149 _]
      frame "空闲" {
      }
      frame "水样测试", Default {
      }
    }
    n170 = case shown="\"空闲\"" w139 {
      selector: w139 -> [w345 _ _ _ _ _ _ _ _ _ _ _]
      tunnel: [w346 "空闲" ("工作状态") "水样测量" ("工作状态") "标样核查" ("工作状态") "零点核查" ("工作状态") "跨度核查" ("工作状态") "空白测试" ("工作状态") "平行样测试" ("工作状态") "加标回收" ("工作状态") "空白校准" ("工作状态") "标样校准" ("工作状态") "初始化" ("工作状态")] -> w138
      frame Default {
        n171 = Format Into String(format string="%d" ("格式字符串"), initial string="未知" ("工作状态"), w345) -> (resulting string=w346:string)  [unwired: 1 in, 1 out]
      }
      frame "空闲" {
      }
      frame "水样测试" {
      }
      frame "标样核查" {
      }
      frame "零点核查" {
      }
      frame "跨度核查" {
      }
      frame "空白测试" {
      }
      frame "平行样测试" {
      }
      frame "加标回收" {
      }
      frame "空白校准" {
      }
      frame "标样校准" {
      }
      frame "初始化（清洗）" {
      }
    }
    n172 = case shown="默认" w137 {
      tunnel: ["" ("字符串") "低量程" ("字符串") "高量程" ("字符串")] -> w136
      frame Default {
      }
      frame 0 {
      }
      frame 1 {
      }
    }
    n173 = global read "VAR总磷总氮全局变量.vi" "序列号"() -> (w141:string)
    n174 = call "告警码字段定义.vi"("告警代码"=w128) -> ("字符串"=w127:string)  [unwired: 8 in, 2 out]
    n175 = call "故障码字段定义.vi"("故障代码"=w126) -> ("字符串"=w125:string)  [unwired: 10 in]
    n176 = Bundle By Name(cluster=T4 {"仪器编号:"="", "工作状态:"="", "运行量程: "="", "数据时间:"=timestamp(0 s since 1904-01-01), "实测值:"="", "数据标识: "="", "仪器时间:"=timestamp(0 s since 1904-01-01), "告警状态: "="", "故障状态:  "="", "因子编码:"=""} ("运行状态"), "仪器编号:"=w141, "仪器时间:"=w140, "工作状态:"=w138, "告警状态:"=w127, "故障状态:"=w125, "运行量程:"=w136, "数据时间:"=w134, "实测值:"=w133, "数据标识:"=w132, "因子编码:"=w131) -> (→"运行状态":T4)
  }
  n177 = call "Create balloon 队列.vi"() -> ("队列输出"=w8:refnum<queue>)  [unwired: 11 in]
  n178 = while {
    shift-right: [w379] -> _
    shift-left: u32 0 ("y") -> [w381]
    stop <- FALSE stop-if-true
    # "密码权限"
    n179 = local read "布尔"() -> (w382:bool)
    n180 = local read "一级权限"() -> (w375:bool)
    n181 = local read "二级权限"() -> (w376:bool)
    n182 = local read "一级权限"() -> (w384:bool)
    n183 = local read "二级权限"() -> (w385:bool)
    n184 = local read "输入密码"() -> (w388:u32)
    n185 = Wait (ms)(milliseconds to wait=u32 1000 ("等待时间（毫秒）")) -> ()  [unwired: 1 out]
    n186 = case shown="假" w382 {
      tunnel: w381 -> [_ w394]
      tunnel: [_ w393] -> w379
      frame False {
      }
      frame True {
        n187 = Increment(x=w394) -> (x+1=w393:u32)
      }
    }
    n188 = global read "VAR总磷总氮全局变量.vi" "MB session in"() -> (w373:refnum<class "MB_Master.lvclass">)
    n189 = Or(x=w384, y=w385) -> (x .or. y?=→"布尔":bool)
    n190 = Equal?(x=w388, y=u32 23506) -> (x = y?=→"二级权限":bool)
    n191 = Or(x=w375, y=w376) -> (x .or. y?=w374:bool)
    n192 = Equal?(x=w388, y=u32 666) -> (x = y?=→"一级权限":bool)
    n193 = property class="MB_Master"(reference=w373) -> ("Properties:Session Valid"=w372:bool)  [unwired: 1 in, 2 out]
    n194 = property on="流程固件" class="Bool"("Visible"=w374) -> ()  [unwired: 2 in, 2 out]
    n195 = property on="启动参数设置" class="Bool"("Visible"=w374) -> ()  [unwired: 2 in, 2 out]
    n196 = Not(x=w372) -> (.not. x?=w371:bool)
    n197 = Greater Or Equal?(x=w379, y=u32 120) -> (x >= y?=w377:bool)
    n198 = property on="模块启用" class="Bool (严格)"("Value"=w371) -> ()  [unwired: 2 in, 2 out]
    n199 = case shown="假" w377 {
      frame False {
      }
      frame True {
        n200 = local write "输入密码"(u32 0 ("输入密码")) -> ()
      }
    }
  }
  n201 = while {
    tunnel: w8 -> [w401]
    shift-right: [w397] -> _
    shift-left: _ -> [w398]
    stop <- FALSE stop-if-true
    n202 = global read "VAR总磷总氮全局变量.vi" "状态告警区"() -> (w395:T7)
    n203 = Wait (ms)(milliseconds to wait=u32 100) -> ()  [unwired: 1 out]
    n204 = Unbundle By Name(w395) -> ("工作状态"=w396:T9, "id"=w403:u16, "日志代码"=w402:u16, "故障代码"=w400:u16, "告警代码"=w399:u16)
    n205 = case shown="\"水样测试\", 默认" w396 {
      tunnel: w403 -> [_ w418]
      tunnel: w402 -> [_ w417]
      tunnel: w401 -> [_ w414]
      tunnel: w400 -> [_ w413]
      tunnel: w399 -> [_ w412]
      tunnel: w398 -> [w406 w411]
      tunnel: [w406 w410] -> w397
      frame "空闲" {
      }
      frame "水样测试", Default {
        n206 = call "id参数转换.vi"("id"=w418) -> ("table输出"=w415:string)  [unwired: 10 in]
        n207 = Add(x=w413, y=w412) -> (x+y=w410:u16)
        n208 = Not Equal?(x=w410, y=w411) -> (x != y?=w408:bool)
        n209 = Not Equal To 0?(x=w410) -> (x != 0?=w409:bool)
        n210 = call "故障告警分析.vi"("告警代码"=w412, "故障代码"=w413, "运行步序"=w417, "参数"=w415) -> ("报警内容"=w416:T19)  [unwired: 6 in, 1 out]
        n211 = And(x=w409, y=w408) -> (x .and. y?=w407:bool)
        n212 = case shown="真" w407 {
          tunnel: w416 -> [_ w427]
          tunnel: w414 -> [_ w426]
          frame False {
          }
          frame True {
            n213 = Unbundle By Name(w427) -> ("参数"=w422:string, "报警内容"=w421:string, "报警分析"=w420:string)
            n214 = Get Date/Time In Seconds() -> (seconds since 1Jan1904=w425:timestamp)
            n215 = Bundle("报警内容"=w421, "报警分析"=w420) -> (w419:cluster{"报警内容":string, "报警分析":string})  [unwired: 1 in]
            n216 = Bundle By Name(cluster=T18 {"时间标识"=timestamp(0 s since 1904-01-01), "设备"="", "日志信息"="", "备注"=""} ("data in"), "时间标识"=w425, "设备"=w422, "日志信息"=w421, "备注"=w420) -> (w424:T18)
            n217 = call "balloon入队列.vi"("报警内容"=w419, "队列"=w426) -> ()  [unwired: 9 in, 1 out]
            n218 = call "总磷总氮报警信息.vi"("data in"=w424) -> ()  [unwired: 10 in, 1 out]
          }
        }
      }
    }
  }
  n219 = Read from Text File(file (use dialog)=w4) -> (text=w5:string)  [unwired: 3 in, 3 out]
  n220 = while {
    shift-right: [w430] -> _
    shift-left: w5 -> [w432]
    tunnel: w4 -> [w429]
    stop <- FALSE stop-if-true
    n221 = Read from Text File(file (use dialog)=w429) -> (text=w430:string)  [unwired: 3 in, 3 out]
    n222 = Not Equal?(x=w432, y=w430) -> (x != y?=w431:bool)
    n223 = Wait (ms)(milliseconds to wait=u32 1000 ("等待时间（毫秒）")) -> ()  [unwired: 1 out]
    n224 = case shown="真" w431 {
      tunnel: w429 -> [_ w434]
      frame False {
      }
      frame True {
        n225 = vi-ref "总磷总氮断电保存全局变量.vi"() -> (w438:refnum<vi>)
        n226 = call <vilib>:"Open Config Data.vi"("configuration file path"=w434) -> ("error out"=w436:errorcluster, "refnum"=w439:T13)  [unwired: 8 in, 1 out]
        n227 = call <userlib>:"Read Panel from INI__ogtk.vi"("error in (no error)"=w436, "VI ref"=w438, "refnum"=w439) -> ("error out"=w435:errorcluster, "refnum out"=w437:T13)  [unwired: 7 in]
        n228 = call <vilib>:"Close Config Data.vi"("error in (no error)"=w435, "refnum"=w437) -> ()  [unwired: 8 in, 2 out]
      }
    }
  }
  n229 = while {
    tunnel: w11 -> [_]
    stop <- FALSE stop-if-true
    # "试剂填充 172 \n管路清洗108\n氨氮92\n总磷131\n总磷海水147\n总氮76\n总氮海水92"
    n230 = global read "VAR总磷总氮全局变量.vi" "状态告警区"() -> (w466:T7)
    n231 = global read "VAR总磷总氮全局变量.vi" "状态告警区"() -> (w464:T7)
    n232 = global read "VAR总磷总氮全局变量.vi" "状态告警区"() -> (w470:T7)
    n233 = global read "VAR总磷总氮全局变量.vi" "状态告警区"() -> (w462:T7)
    n234 = Wait (ms)(milliseconds to wait=u32 1000 ("等待时间（毫秒）")) -> ()  [unwired: 1 out]
    n235 = Unbundle By Name(w470) -> ("id"=w467:u16, "flowid"=w469:u16, "量程"=w468:u16, "工作状态"=w455:T9, "F0"=→"F0":sgl, "F1"=→"F1":sgl, "F2"=→"F2":sgl, "F3"=→"F3":sgl, "ADC"=→"ADC":sgl, "总磷控温温度1"=→"温度1":sgl, "营养盐控温温度2"=→"温度2":sgl)
    n236 = Unbundle By Name(w462) -> ("日志代码"=w461:u16)
    n237 = Unbundle By Name(w466) -> ("日志代码"=w458:u16)
    n238 = Unbundle By Name(w464) -> ("工作状态"=w450:T9, "id"=w451:u16)
    n239 = case shown="\"空闲\"" w450 {
      frame "空闲" {
        n240 = local write "数组"(string[] [] ("数组")) -> ()
      }
      frame "水样测试", Default {
      }
    }
    n241 = feedback-in #2(w458) -> ()
    n242 = feedback #2(w458) -> (w475:u16)
    n243 = feedback #3(w461) -> (w463:u16)
    n244 = feedback-in #3(w461) -> ()
    n245 = Not Equal To 0?(x=w450) -> (x != 0?=w448:bool)
    n246 = Subtract(x=w458, y=1) -> (x-y=→"多列列表框":i32)
    n247 = Not Equal?(x=w458, y=w475) -> (x != y?=w474:bool)
    n248 = call <vilib>:"Boolean Crossing PtByPt.vi"("direction"=enum16{"either", "false-true", "true-false"}."false-true", "input"=w448) -> ("crossing"=w452:bool)  [unwired: 1 in]
    n249 = call <vilib>:"Boolean Crossing PtByPt.vi"("direction"=enum16{"either", "false-true", "true-false"}."true-false", "input"=w448) -> ("crossing"=w447:bool)  [unwired: 1 in]
    n250 = Not Equal To 0?(x=w455) -> (x != 0?=w472:bool)
    n251 = case shown="假" w474 {
      tunnel: w458 -> [_ w611]
      frame False {
      }
      frame True {
        n252 = Subtract(x=w611, y=1) -> (x-y=w609:i32)
        n253 = Subtract(x=w609, y=5) -> (x-y=w613:i32)
        n254 = Greater Or Equal To 0?(x=w613) -> (x >= 0?=w612:bool)
        n255 = property on="多列列表框" class="MCListbox (严格)"() -> (error out=w617:errorcluster, "TopLeft"=w618:T22)  [unwired: 2 in, 1 out]
        n256 = Select(t=w613, s=w612, f=0) -> (s? t:f=w614:i32)
        n257 = Bundle By Name(cluster=w618, "Row"=w614) -> (w619:T22)
        n258 = property on="多列列表框" class="MCListbox (严格)"(error in=w617, "TopLeft"=w619) -> ()  [unwired: 1 in, 2 out]
      }
    }
    n259 = case shown="真" w452 {
      tunnel: w450 -> [_ w501]
      tunnel: w451 -> [_ w498]
      frame False {
      }
      frame True {
        n260 = case shown="\"空闲\", 默认" w501 {
          tunnel: [_ "【水样测试】" ("字符串") "【标样核查】" ("字符串") "【零点核查】" ("字符串") "【跨度核查】" ("字符串") "【空白测试】" ("字符串") "【平行样测试】" ("字符串") "【加标回收】" ("字符串") "【空白校准】" ("字符串") "【标样校准】" ("字符串")] -> w506
          frame "空闲", Default {
          }
          frame "水样测试" {
          }
          frame "标样核查" {
          }
          frame "零点核查" {
          }
          frame "跨度核查" {
          }
          frame "空白测试" {
          }
          frame "平行样测试" {
          }
          frame "加标回收" {
          }
          frame "空白校准" {
          }
          frame "标样校准" {
          }
        }
        n261 = call "id参数转换.vi"("id"=w498) -> ("table输出"=w497:string)  [unwired: 10 in]
        n262 = Concatenate Strings("-->>" ("字符串"), w506, "启动" ("字符串")) -> (w505:string)
        n263 = Get Date/Time In Seconds() -> (seconds since 1Jan1904=w503:timestamp)
        n264 = Bundle By Name(cluster=T21 {"时间标识"=timestamp(0 s since 1904-01-01), "设备"="", "日志信息"="", "流程参数"=""} ("data in"), "时间标识"=w503, "设备"=w497, "日志信息"=w505) -> (w502:T21)
        n265 = call "总磷总氮操作日志.vi"("data in"=w502) -> ()  [unwired: 11 in]
      }
    }
    n266 = case shown="真" w447 {
      tunnel: w450 -> [_ w482]
      tunnel: w451 -> [_ w479]
      frame False {
      }
      frame True {
        n267 = case shown="\"水样测试\"" w482 {
          tunnel: [_ "【水样测试】" ("字符串") "【标样核查】" ("字符串") "【零点核查】" ("字符串") "【跨度核查】" ("字符串") "【空白测试】" ("字符串") "【平行样测试】" ("字符串") "【加标回收】" ("字符串") "【空白校准】" ("字符串") "【标样校准】" ("字符串")] -> w487
          frame "空闲", Default {
          }
          frame "水样测试" {
          }
          frame "标样核查" {
          }
          frame "零点核查" {
          }
          frame "跨度核查" {
          }
          frame "空白测试" {
          }
          frame "平行样测试" {
          }
          frame "加标回收" {
          }
          frame "空白校准" {
          }
          frame "标样校准" {
          }
        }
        n268 = call "id参数转换.vi"("id"=w479) -> ("table输出"=w478:string)  [unwired: 10 in]
        n269 = Concatenate Strings("-->>" ("字符串"), w487, "停止" ("字符串")) -> (w486:string)
        n270 = Get Date/Time In Seconds() -> (seconds since 1Jan1904=w484:timestamp)
        n271 = Bundle By Name(cluster=T21 {"时间标识"=timestamp(0 s since 1904-01-01), "设备"="", "日志信息"="", "流程参数"=""} ("data in"), "时间标识"=w484, "设备"=w478, "日志信息"=w486) -> (w483:T21)
        n272 = call "总磷总氮操作日志.vi"("data in"=w483) -> ()  [unwired: 11 in]
      }
    }
    n273 = call <vilib>:"Boolean Crossing PtByPt.vi"("input"=w472) -> ("crossing"=w454:bool)  [unwired: 2 in]
    n274 = Bundle By Name(cluster=T20 {"启动模式"=enum."跨度核查", "启动参数"=1, "量程"=enum."低量程"} ("参数簇"), "启动参数"=w467, "启动模式"=w469, "量程"=w468) -> (w465:T20)
    n275 = First Call?() -> (First Call?: T/F=w473:bool)
    n276 = Or(x=w454, y=w473) -> (x .or. y?=w471:bool)
    n277 = while {
      tunnel: w471 -> [w597]
      tunnel: w465 -> [w596]
      shift-right: [w591] -> _
      shift-left: _ -> [w593]
      shift-right: [w592] -> _
      shift-left: _ -> [w594]
      shift-right: ["流程路径"] -> _
      shift-left: _ -> [w589]
      stop <- TRUE stop-if-true
      n278 = Not Equal?(x=w589, y="流程路径") -> (x != y?=w587:bool)
      n279 = Or(x=w597, y=w587) -> (x .or. y?=w588:bool)
      n280 = case shown="真" w588 {
        tunnel: [w599 w607] -> w592
        tunnel: [w598 w606] -> w591
        tunnel: w596 -> [_ w601]
        tunnel: w594 -> [w599 _]
        tunnel: w593 -> [w598 _]
        tunnel: "流程路径" -> [_ w600]
        frame False {
        }
        frame True {
          n281 = call "斯坦道XML解析.vi"("添加的路径"=w600, "参数簇"=w601) -> ("步骤时间"=w602:string[], "步骤名"=w604:string[])  [unwired: 8 in]
          n282 = Build Array(w604, w602) -> (w603:string[][])
          n283 = for {
            tunnel: w604 -> [_] mode=indexing
            tunnel: [w608] -> w605 mode=indexing
            i -> [w608]
          }
          n284 = Transpose 2D Array(2D array=w603) -> (transposed array=w606:string[][])
          n285 = Number To Decimal String(number=w605) -> (decimal integer string=w607:string[])  [unwired: 1 in]
        }
      }
      n286 = property on="多列列表框" class="MCListbox (严格)"("ItemNames"=w591, "RowHdrs[]"=w592) -> ()  [unwired: 2 in, 2 out]
    }
    n287 = Not Equal?(x=w461, y=w463) -> (x != y?=w460:bool)
    n288 = case shown="真" w460 {
      frame False {
      }
      frame True {
        n289 = property on="多列列表框" class="MCListbox (严格)"() -> ("ItemNames"=w521:string[][], "Value"=w517:i32)  [unwired: 2 in, 2 out]
        n290 = Index Array(array=w521, index (row)=w517) -> (element=w520:string[])  [unwired: 1 in]
        n291 = Index Array(array=w520) -> (element=w519:string)  [unwired: 1 in]
        n292 = call "过滤筛选流程.vi"("字符串"=w519) -> ("匹配后偏移量"=w518:i32)  [unwired: 10 in]
        n293 = case shown="默认" w518 {
          tunnel: w519 -> [w523 _]
          tunnel: w517 -> [w522 _]
          frame Default {
            n294 = case shown="默认" w523 {
              selector: w523 -> [w529 w536]
              tunnel: [w529 w536] -> w525
              tunnel: [string[] [] ("数组") w531] -> w524
              tunnel: w522 -> [_ w535]
              frame "读数" {
              }
              frame Default {
                n295 = Equal?(x=w535, y=1) -> (x = y?=w533:bool)
                n296 = Select(t=string[] [], s=w533, f="数组") -> (s? t:f=w531:string[])
              }
            }
            n297 = for {
              N: 1 -> [_]
              tunnel: w525 -> [w538]
              shift-right: [w537] -> w526
              shift-left: w524 -> [w539]
              n298 = Search 1D Array(1D array=w539, element=w538) -> (index of element=w542:i32)  [unwired: 1 in]
              n299 = Format Into String(format string="%s" ("格式字符串"), w538) -> (resulting string=w543:string)  [unwired: 2 in, 1 out]
              n300 = Equal?(x=w542, y=-1) -> (x = y?=w540:bool)
              n301 = case shown="真" w540 {
                tunnel: w543 -> [_ w553]
                tunnel: w539 -> [w545 w557]
                tunnel: w538 -> [_ w556]
                tunnel: [w545 w555] -> w537
                frame False {
                }
                frame True {
                  n302 = case shown="\"结束\"" w553 {
                    selector: w553 -> [w580 w583 w586]
                    tunnel: [w580 w582 w585] -> w552
                    frame Default {
                    }
                    frame "初始化" {
                      n303 = Concatenate Strings("-->>" ("字符串"), w583) -> (w582:string)
                    }
                    frame "结束" {
                      n304 = Concatenate Strings("-->>" ("字符串"), w586) -> (w585:string)
                    }
                  }
                  n305 = Insert Into Array(array=w557, new element=w556) -> (w555:string[])  [unwired: 1 in]
                  n306 = global read "VAR总磷总氮全局变量.vi" "状态告警区"() -> (w551:T7)
                  n307 = Unbundle By Name(w551) -> ("工作状态"=w550:T9)
                  n308 = case shown="\"水样测试\"" w550 {
                    tunnel: [_ "【水样测试】" ("字符串") "【标样核查】" ("字符串") "【零点核查】" ("字符串") "【跨度核查】" ("字符串") "【空白测试】" ("字符串") "【平行样测试】" ("字符串") "【加标回收】" ("字符串") "【空白校准】" ("字符串") "【标样校准】" ("字符串")] -> w548
                    frame "空闲", Default {
                    }
                    frame "水样测试" {
                    }
                    frame "标样核查" {
                    }
                    frame "零点核查" {
                    }
                    frame "跨度核查" {
                    }
                    frame "空白测试" {
                    }
                    frame "平行样测试" {
                    }
                    frame "加标回收" {
                    }
                    frame "空白校准" {
                    }
                    frame "标样校准" {
                    }
                  }
                  n309 = global read "VAR总磷总氮全局变量.vi" "状态告警区"() -> (w570:T7)
                  n310 = global read "VAR总磷总氮全局变量.vi" "状态告警区"() -> (w567:T7)
                  n311 = Unbundle By Name(w567) -> ("F0"=w564:sgl, "F1"=w563:sgl, "F2"=w562:sgl, "F3"=w561:sgl, "id"=w560:u16, "flowid"=w559:u16, "量程"=w558:u16)
                  n312 = Unbundle By Name(w570) -> ("id"=w547:u16)
                  n313 = call "id参数转换.vi"("id"=w547) -> ("table输出"=w546:string)  [unwired: 10 in]
                  n314 = Concatenate Strings(w548, w552) -> (w549:string)
                  n315 = Format Into String(format string="F0=%#f,F1=%#f,F2=%#f,F3=%#f,Flow=%d-%-d-%-d" ("格式字符串"), w564, w563, w562, w561, w560, w559, w558) -> (resulting string=w565:string)  [unwired: 2 in, 1 out]
                  n316 = Get Date/Time In Seconds() -> (seconds since 1Jan1904=w568:timestamp)
                  n317 = Bundle By Name(cluster=T21 {"时间标识"=timestamp(0 s since 1904-01-01), "设备"="", "日志信息"="", "流程参数"=""} ("data in"), "时间标识"=w568, "设备"=w546, "日志信息"=w549, "流程参数"=w565) -> (w569:T21)
                  n318 = call "总磷总氮操作日志.vi"("data in"=w569) -> ()  [unwired: 11 in]
                }
              }
            }
            n319 = local write "数组"(w526) -> ()
          }
          frame -1 {
          }
        }
      }
    }
  }
  n320 = call "设置模块队列名.vi"() -> ("Msg"=w2:string)  [unwired: 5 in]
  n321 = Obtain Queue(name (unnamed)=w6, element data type=cluster{"命令":string, "data":variant} {"命令"="", "data"=variant}) -> (queue out=w7:refnum<queue>)  [unwired: 3 in, 2 out]
  n322 = Obtain Notifier(name (unnamed)=w2, notification data type=FALSE) -> (notifier out=w1:refnum<notifier>)  [unwired: 2 in, 2 out]
  n323 = control-ref of="测量模式下拉列表"() -> (w14:refnum<vi>)
  n324 = while {
    tunnel: w7 -> [w624]
    tunnel: [w622] -> _
    stop <- FALSE stop-if-true
    # "定时更新"
    n325 = Get Queue Status(queue=w624) -> (queue out=w621:refnum<queue>, # elements in queue=w620:i32)  [unwired: 2 in, 6 out]
    n326 = Wait (ms)(milliseconds to wait=u32 1000 ("等待时间（毫秒）")) -> ()  [unwired: 1 out]
    n327 = case shown="0" w620 {
      tunnel: w621 -> [_ w632]
      tunnel: [_ w630] -> w622
      frame Default {
      }
      frame 0 {
        n328 = global read "VAR总磷总氮全局变量.vi" "启动队列名称"() -> (w628:cluster{"String":string, "Value":u16}[])
        n329 = Index Array(array=w628) -> (element=w627:cluster{"String":string, "Value":u16})  [unwired: 1 in]
        n330 = Unbundle By Name(w627) -> ("Value"=w626:u16)
        n331 = call "总磷总氮版本号读取.vi"("Slave ID"=w626) -> ("error out"=w630:errorcluster, "固件版本号"=→"固件版本号":string)  [unwired: 9 in]
        n332 = Bundle By Name(cluster=cluster{"命令":string, "data":variant} {"命令"="", "data"=variant} ("元素"), "命令"="读序列号", "data"=w626) -> (w631:cluster{"命令":string, "data":variant})
        n333 = Enqueue Element(queue=w632, element=w631) -> ()  [unwired: 2 in, 3 out]
      }
    }
  }
  n334 = while {
    tunnel: w7 -> [w640]
    stop <- FALSE stop-if-true
    n335 = Get Queue Status(queue=w640) -> (queue out=w638:refnum<queue>, # elements in queue=w637:i32)  [unwired: 2 in, 6 out]
    n336 = Wait (ms)(milliseconds to wait=u32 1000 ("等待时间（毫秒）")) -> ()  [unwired: 1 out]
    n337 = case shown="0" w637 {
      tunnel: w638 -> [_ w656]
      frame Default {
      }
      frame 0 {
        n338 = global read "VAR总磷总氮全局变量.vi" "启动队列名称"() -> (w645:cluster{"String":string, "Value":u16}[])
        n339 = for {
          tunnel: [w674] -> w646 mode=indexing
          tunnel: w645 -> [w675] mode=indexing
          n340 = Unbundle By Name(w675) -> ("Value"=w674:u16)
        }
        n341 = global read "VAR总磷总氮全局变量.vi" "状态告警区"() -> (w648:T7)
        n342 = Unbundle By Name(w648) -> ("系统时间"=w655:timestamp, "工作状态"=w647:T9)
        n343 = for {
          tunnel: w647 -> [w660]
          shift-right: [w661] -> w649
          shift-left: w656 -> [w663]
          tunnel: w646 -> [w657] mode=indexing
          n344 = Equal?(x=w660, y=T9."空闲") -> (x = y?=w658:bool)
          n345 = Bundle By Name(cluster=cluster{"命令":string, "data":variant} {"命令"="", "data"=variant} ("元素"), "命令"="读状态告警区", "data"=w657) -> (w665:cluster{"命令":string, "data":variant})
          n346 = Enqueue Element(queue=w663, element=w665) -> (queue out=w662:refnum<queue>)  [unwired: 2 in, 2 out]
          n347 = case shown="真" w658 {
            tunnel: w662 -> [w667 w670]
            tunnel: w657 -> [_ w669]
            tunnel: [w667 w668] -> w661
            frame False {
            }
            frame True {
              n348 = Bundle By Name(cluster=cluster{"命令":string, "data":variant} {"命令"="", "data"=variant} ("元素"), "命令"="读测量数据区", "data"=w669) -> (w672:cluster{"命令":string, "data":variant})
              n349 = Enqueue Element(queue=w670, element=w672) -> (queue out=w668:refnum<queue>)  [unwired: 2 in, 2 out]
            }
          }
        }
        n350 = Get Date/Time In Seconds() -> (seconds since 1Jan1904=w654:timestamp)
        n351 = Subtract(x=w654, y=w655) -> (x-y=w653:dbl)
        n352 = Absolute Value(x=w653) -> (abs(x)=w652:dbl)
        n353 = Greater Or Equal?(x=w652, y=120.0) -> (x >= y?=w650:bool)
        n354 = case shown="真" w650 {
          tunnel: w649 -> [_ w677]
          frame False {
          }
          frame True {
            n355 = call "总磷总氮启动命令.vi"("参数"=T23 {"站号"=3, "量程切换"=enum."AUTO", "控制命令"=enum."校时", "模式设置"=enum."待机", "测量间隔"=0}) -> ("启动命令"=w676:cluster{"命令":string, "data":variant})  [unwired: 10 in]
            n356 = Enqueue Element(queue=w677, element=w676) -> ()  [unwired: 2 in, 3 out]
          }
        }
      }
    }
    n357 = global read "总磷总氮断电保存全局变量.vi" "流程路径"() -> (w639:path)
    n358 = local write "流程路径"(w639) -> ()
    n359 = global read "总磷总氮断电保存全局变量.vi" "MB通信方式选择"() -> (w636:enum16{"串口", "TCP"})
    n360 = case shown="\"串口\", 默认" w636 {
      tunnel: [w643 w644] -> w635
      frame "串口", Default {
        n361 = global read "总磷总氮断电保存全局变量.vi" "VISA Resource"() -> (w643:refnum<visa-resource-name>)
      }
      frame "TCP" {
        n362 = global read "总磷总氮断电保存全局变量.vi" "IP"() -> (w644:string)
      }
    }
    "字符串 2" <- w635
  }
  n363 = control-ref of="量程参数读取"() -> (w12:refnum<vi>)
  n364 = control-ref of="参数下拉列表"() -> (w15:refnum<vi>)
  n365 = control-ref of="量程下拉列表"() -> (w16:refnum<vi>)
  n366 = control-ref of="公式"() -> (w13:refnum<vi>)
  n367 = while {
    tunnel: w7 -> [w685]
    tunnel: w16 -> [w684]
    tunnel: w15 -> [w683]
    tunnel: w14 -> [w682]
    tunnel: w13 -> [w681]
    tunnel: w12 -> [w680]
    tunnel: w1 -> [w679]
    stop <- FALSE stop-if-true
    n368 = event shown="[15] \"停止\": 值改变" {
      selector: _ -> [_ _ _ _ _ _ _ _ _ _ _ _ _ _ _ _ _ _ _ _ _ _ _]
      dyn-events: _ -> [_ _ _ _ _ _ _ _ _ _ _ _ _ _ _ _ _ _ _ _ _ _ _]
      timeout: _ -> [_ _ _ _ _ _ _ _ _ _ _ _ _ _ _ _ _ _ _ _ _ _ _]
      tunnel: w685 -> [_ _ _ _ _ w705 w731 _ _ _ _ _ _ w828 _ w837 _ _ _ _ _ _ _]
      tunnel: w684 -> [_ _ _ _ _ _ _ _ w751 _ _ _ _ _ _ _ _ _ _ w853 _ _ _]
      tunnel: w683 -> [_ _ _ _ _ _ _ _ w755 _ _ _ w806 _ _ _ _ _ _ w851 _ w904 w911]
      tunnel: w682 -> [_ _ _ _ _ _ _ _ w753 _ _ _ _ _ _ _ _ _ _ w852 _ _ _]
      tunnel: w681 -> [_ _ _ _ _ _ _ _ _ _ _ _ _ _ _ _ _ _ _ w847 _ _ _]
      tunnel: w680 -> [_ _ _ _ _ _ _ _ _ _ _ _ _ _ _ _ _ _ _ _ _ w902 _]
      tunnel: [_ _ _ w691 _ _ _ _ _ _ _ _ _ _ _ _ _ _ _ _ _ _ _] -> _
      tunnel: w679 -> [_ _ _ _ _ _ _ _ _ _ _ _ _ _ _ w833 _ _ _ _ _ _ _]
      event Timeout {
        n369 = event-data() -> ()  [unwired: 1 in, 3 out]
      }
      event "启动参数设置": Value Change {
        n370 = event-data() -> ()  [unwired: 1 in, 6 out]
        n371 = call "启动参数设置.vi"() -> ()  [unwired: 12 in]
      }
      event "布尔": Mouse Down {
        n372 = event-data() -> ("CtlRef"=w688:refnum<vi>)  [unwired: 1 in, 5 out]
        n373 = property class="Bool (严格)"(reference=w688) -> ("Value"=w687:bool)  [unwired: 1 in, 2 out]
        n374 = case shown="真" w687 {
          frame False {
            n375 = call "密码键盘.vi"() -> ("NewNumber"=→"输入密码":dbl)  [unwired: 1 in]
          }
          frame True {
            n376 = local write "输入密码"(u32 0 ("输入密码")) -> ()
          }
        }
      }
      event "测量模式下拉列表", "量程下拉列表", "参数下拉列表": Value Change {
        n377 = event-data() -> ()  [unwired: 1 in, 6 out]
        n378 = local read "测量模式下拉列表"() -> (w694:enum16{"水样测量", "零点核查", "跨度核查", "标样核查", "加标回收"})
        n379 = local read "参数下拉列表"() -> (w693:enum16{"COD", "氨氮", "总氮", "总磷"})
        n380 = local read "量程下拉列表"() -> (w695:enum16{"低量程", "高量程"})
        n381 = Bundle("参数下拉列表"=w693, "测量模式下拉列表"=w694, "量程下拉列表"=w695) -> (w692:T24)  [unwired: 1 in]
        n382 = property on="曲线模型" class="曲线模型 (严格)"("属性"=w692) -> (error out=w691:errorcluster)  [unwired: 2 in, 1 out]
      }
      event "流程固件": Value Change {
        n383 = event-data() -> ()  [unwired: 1 in, 6 out]
        n384 = call "流程固件设置对话框.vi"() -> ()  [unwired: 12 in]
      }
      event "串口设置": Value Change {
        n385 = event-data() -> ()  [unwired: 1 in, 6 out]
        n386 = global read "总磷总氮断电保存全局变量.vi" "MB通信方式选择"() -> (w696:enum16{"串口", "TCP"})
        n387 = global read "总磷总氮断电保存全局变量.vi" "VISA Resource"() -> (w702:refnum<visa-resource-name>)
        n388 = global read "总磷总氮断电保存全局变量.vi" "PORT"() -> (w700:string)
        n389 = global read "总磷总氮断电保存全局变量.vi" "IP"() -> (w701:string)
        n390 = call "串口配置.vi"("PORT"=w700, "IP"=w701, "MB通信方式选择"=w696, "请选择串口:"=w702) -> ("PORT 2"=w698:string, "IP 2"=w699:string, "确认 2"=w703:bool, "VISA资源名称 2"=w704:refnum<visa-resource-name>, "MB通信方式选择 2"=w697:enum16{"串口", "TCP"})  [unwired: 3 in]
        n391 = case shown="真" w703 {
          tunnel: w704 -> [_ w710]
          tunnel: w705 -> [_ w709]
          tunnel: w699 -> [_ w708]
          tunnel: w698 -> [_ w707]
          tunnel: w697 -> [_ w706]
          frame False {
          }
          frame True {
            n392 = flat-sequence {
              tunnel: w710 -> [w715]
              tunnel: w709 -> [w716]
              tunnel: w708 -> [w714]
              tunnel: w707 -> [w713]
              tunnel: w706 -> [w712]
              frame #0 {
                n393 = global write "总磷总氮断电保存全局变量.vi" "IP"(w714) -> ()
                n394 = global write "总磷总氮断电保存全局变量.vi" "PORT"(w713) -> ()
                n395 = global write "总磷总氮断电保存全局变量.vi" "VISA Resource"(w715) -> ()
                n396 = global write "总磷总氮断电保存全局变量.vi" "MB通信方式选择"(w712) -> ()
                n397 = Flush Queue(queue=w716) -> (queue out=w711:refnum<queue>)  [unwired: 1 in, 2 out]
                n398 = Enqueue Element(queue=w711, element=cluster{"命令":string, "data":variant} {"命令"="启用模块", "data"=variant} ("元素")) -> ()  [unwired: 2 in, 3 out]
              }
              frame #1 {
                n399 = call "配置文件路径.vi"() -> ("appended path"=w718:path)  [unwired: 11 in]
                n400 = call <vilib>:"Open Config Data.vi"("configuration file path"=w718) -> ("error out"=w726:errorcluster, "refnum"=w729:T13)  [unwired: 8 in, 1 out]
                n401 = vi-ref "总磷总氮断电保存全局变量.vi"() -> (w728:refnum<vi>)
                n402 = call <userlib>:"Write Panel to INI__ogtk.vi"("error in (no error)"=w726, "VI ref"=w728, "refnum"=w729) -> ("error out"=w725:errorcluster, "refnum out"=w727:T13)  [unwired: 7 in]
                n403 = call <vilib>:"Close Config Data.vi"("error in (no error)"=w725, "refnum"=w727) -> ("error out"=w720:errorcluster, "file path"=w719:path)  [unwired: 8 in]
                n404 = Open/Create/Replace File(file path (use dialog)=w719, error in=w720) -> (refnum out=w723:refnum<file>, error out=w724:errorcluster)  [unwired: 4 in, 1 out]
                n405 = Flush File(refnum=w723, error in=w724) -> (refnum out=w722:refnum<file>, error out=w721:errorcluster)
                n406 = Close File(refnum=w722, error in=w721) -> ()  [unwired: 2 out]
              }
            }
          }
        }
      }
      event "模块启用": Value Change {
        n407 = event-data() -> ("OldVal"=w732:bool)  [unwired: 1 in, 5 out]
        n408 = Flush Queue(queue=w731) -> (queue out=w730:refnum<queue>)  [unwired: 1 in, 2 out]
        n409 = case shown="假" w732 {
          tunnel: w730 -> [w733 w735]
          frame False {
            n410 = Enqueue Element(queue=w733, element=cluster{"命令":string, "data":variant} {"命令"="停用模块", "data"=variant} ("元素")) -> ()  [unwired: 2 in, 3 out]
          }
          frame True {
            n411 = Enqueue Element(queue=w735, element=cluster{"命令":string, "data":variant} {"命令"="启用模块", "data"=variant} ("元素")) -> ()  [unwired: 2 in, 3 out]
          }
        }
      }
      event "流程路径": Value Change {
        n412 = event-data() -> ()  [unwired: 1 in, 6 out]
        n413 = flat-sequence {
          frame #0 {
            n414 = local read "流程路径"() -> (w737:path)
            n415 = global write "总磷总氮断电保存全局变量.vi" "流程路径"(w737) -> ()
          }
          frame #1 {
            n416 = call "配置文件路径.vi"() -> ("appended path"=w738:path)  [unwired: 11 in]
            n417 = call <vilib>:"Open Config Data.vi"("configuration file path"=w738) -> ("error out"=w746:errorcluster, "refnum"=w749:T13)  [unwired: 8 in, 1 out]
            n418 = vi-ref "总磷总氮断电保存全局变量.vi"() -> (w748:refnum<vi>)
            n419 = call <userlib>:"Write Panel to INI__ogtk.vi"("error in (no error)"=w746, "VI ref"=w748, "refnum"=w749) -> ("error out"=w745:errorcluster, "refnum out"=w747:T13)  [unwired: 7 in]
            n420 = call <vilib>:"Close Config Data.vi"("error in (no error)"=w745, "refnum"=w747) -> ("error out"=w740:errorcluster, "file path"=w739:path)  [unwired: 8 in]
            n421 = Open/Create/Replace File(file path (use dialog)=w739, error in=w740) -> (refnum out=w743:refnum<file>, error out=w744:errorcluster)  [unwired: 4 in, 1 out]
            n422 = Flush File(refnum=w743, error in=w744) -> (refnum out=w742:refnum<file>, error out=w741:errorcluster)
            n423 = Close File(refnum=w742, error in=w741) -> ()  [unwired: 2 out]
          }
        }
      }
      event "公式一键写入": Value Change {
        n424 = event-data() -> ()  [unwired: 1 in, 6 out]
        n425 = property class="Enum (严格)"(reference=w755) -> ("Value"=w754:enum16{"COD", "氨氮", "总氮", "总磷"})  [unwired: 1 in, 2 out]
        n426 = property class="Enum (严格)"(reference=w753) -> ("Value"=w752:enum16{"水样测量", "零点核查", "跨度核查", "标样核查", "加标回收"})  [unwired: 1 in, 2 out]
        n427 = property class="Enum (严格)"(reference=w751) -> ("Value"=w750:enum16{"低量程", "高量程"})  [unwired: 1 in, 2 out]
        n428 = local read "公式"() -> (w757:cluster{"X^2":dbl, "X":dbl, "b":dbl})
        n429 = call "公式复合写入.vi"("公式"=w757, "量程下拉列表"=w750, "测量模式下拉列表"=w752, "参数下拉列表"=w754) -> ("模型复制"=w756:T25)  [unwired: 7 in]
        n430 = invoke on="曲线模型" class="曲线模型 (严格)" method="模型复制.vi"("模型复制"=w756) -> ()  [unwired: 3 in, 4 out]
      }
      event "曲线模型": Value Change {
        n431 = event-data() -> ()  [unwired: 1 in, 6 out]
        n432 = Unbundle By Name("曲线模型") -> ("X^2"=w761:dbl, "X"=w760:dbl, "B"=w759:dbl)
        n433 = Bundle("X^2"=w761, "X"=w760, "B"=w759) -> (w758:cluster{"X^2":dbl, "X":dbl, "B":dbl})  [unwired: 1 in]
        n434 = local write "公式"(w758) -> ()
      }
      event "质控参数设置": Value Change {
        n435 = event-data() -> ()  [unwired: 1 in, 6 out]
        n436 = global read "总磷总氮断电保存全局变量.vi" "质控参数设置"() -> (w765:T26)
        n437 = call "总磷总氮质控参数设置.vi"("质控参数设置"=w765) -> ("质控参数设置 2"=w763:T26, "check？"=w764:bool)  [unwired: 9 in]
        n438 = case shown="真" w764 {
          tunnel: w765 -> [_ w767]
          tunnel: w763 -> [_ w766]
          frame False {
          }
          frame True {
            n439 = flat-sequence {
              tunnel: w767 -> [_]
              tunnel: w766 -> [w768]
              frame #0 {
                n440 = global write "总磷总氮断电保存全局变量.vi" "质控参数设置"(w768) -> ()
              }
              frame #1 {
                n441 = call "配置文件路径.vi"() -> ("appended path"=w769:path)  [unwired: 11 in]
                n442 = call <vilib>:"Open Config Data.vi"("configuration file path"=w769) -> ("error out"=w777:errorcluster, "refnum"=w780:T13)  [unwired: 8 in, 1 out]
                n443 = vi-ref "总磷总氮断电保存全局变量.vi"() -> (w779:refnum<vi>)
                n444 = call <userlib>:"Write Panel to INI__ogtk.vi"("error in (no error)"=w777, "VI ref"=w779, "refnum"=w780) -> ("error out"=w776:errorcluster, "refnum out"=w778:T13)  [unwired: 7 in]
                n445 = call <vilib>:"Close Config Data.vi"("error in (no error)"=w776, "refnum"=w778) -> ("error out"=w771:errorcluster, "file path"=w770:path)  [unwired: 8 in]
                n446 = Open/Create/Replace File(file path (use dialog)=w770, error in=w771) -> (refnum out=w774:refnum<file>, error out=w775:errorcluster)  [unwired: 4 in, 1 out]
                n447 = Flush File(refnum=w774, error in=w775) -> (refnum out=w773:refnum<file>, error out=w772:errorcluster)
                n448 = Close File(refnum=w773, error in=w772) -> ()  [unwired: 2 out]
              }
            }
          }
        }
      }
      event "仪器参数": Value Change {
        n449 = event-data() -> ()  [unwired: 1 in, 6 out]
        n450 = global read "总磷总氮断电保存全局变量.vi" "COD仪器参数"() -> (w786:T27)
        n451 = global read "总磷总氮断电保存全局变量.vi" "氨氮仪器参数"() -> (w785:T27)
        n452 = global read "总磷总氮断电保存全局变量.vi" "总氮仪器参数"() -> (w784:T27)
        n453 = global read "总磷总氮断电保存全局变量.vi" "总磷仪器参数"() -> (w783:T27)
        n454 = Bundle("COD仪器参数"=w786, "氨氮仪器参数"=w785, "总氮仪器参数"=w784, "总磷仪器参数"=w783) -> (w782:T28)  [unwired: 1 in]
        n455 = call "仪器参数设置.vi"("仪器参数"=w782) -> ("仪器参数 2"=w781:T28, "check？"=w787:bool)  [unwired: 9 in]
        n456 = case shown="真" w787 {
          tunnel: w781 -> [_ w788]
          frame False {
          }
          frame True {
            n457 = flat-sequence {
              tunnel: w788 -> [w793]
              frame #0 {
                n458 = Unbundle By Name(w793) -> ("COD仪器参数"=w791:T27, "氨氮仪器参数"=w790:T27, "总氮仪器参数"=w792:T27, "总磷仪器参数"=w789:T27)
                n459 = global write "总磷总氮断电保存全局变量.vi" "COD仪器参数"(w791) -> ()
                n460 = global write "总磷总氮断电保存全局变量.vi" "氨氮仪器参数"(w790) -> ()
                n461 = global write "总磷总氮断电保存全局变量.vi" "总氮仪器参数"(w792) -> ()
                n462 = global write "总磷总氮断电保存全局变量.vi" "总磷仪器参数"(w789) -> ()
              }
              frame #1 {
                n463 = call "配置文件路径.vi"() -> ("appended path"=w794:path)  [unwired: 11 in]
                n464 = call <vilib>:"Open Config Data.vi"("configuration file path"=w794) -> ("error out"=w802:errorcluster, "refnum"=w805:T13)  [unwired: 8 in, 1 out]
                n465 = vi-ref "总磷总氮断电保存全局变量.vi"() -> (w804:refnum<vi>)
                n466 = call <userlib>:"Write Panel to INI__ogtk.vi"("error in (no error)"=w802, "VI ref"=w804, "refnum"=w805) -> ("error out"=w801:errorcluster, "refnum out"=w803:T13)  [unwired: 7 in]
                n467 = call <vilib>:"Close Config Data.vi"("error in (no error)"=w801, "refnum"=w803) -> ("error out"=w796:errorcluster, "file path"=w795:path)  [unwired: 8 in]
                n468 = Open/Create/Replace File(file path (use dialog)=w795, error in=w796) -> (refnum out=w799:refnum<file>, error out=w800:errorcluster)  [unwired: 4 in, 1 out]
                n469 = Flush File(refnum=w799, error in=w800) -> (refnum out=w798:refnum<file>, error out=w797:errorcluster)
                n470 = Close File(refnum=w798, error in=w797) -> ()  [unwired: 2 out]
              }
            }
          }
        }
      }
      event "测试量程配置": Value Change {
        n471 = event-data() -> ()  [unwired: 1 in, 6 out]
        n472 = flat-sequence {
          tunnel: w806 -> [w809]
          frame #0 {
            n473 = property class="Enum (严格)"(reference=w809) -> ("Value"=w808:enum16{"COD", "氨氮", "总氮", "总磷"})  [unwired: 1 in, 2 out]
            n474 = case shown="默认" w808 {
              tunnel: "测试量程配置" -> [_ w810 w811 w812 w813]
              frame Default {
              }
              frame "COD" {
                n475 = global write "总磷总氮断电保存全局变量.vi" "COD自动测试量程配置"(w810) -> ()
              }
              frame "氨氮" {
                n476 = global write "总磷总氮断电保存全局变量.vi" "氨氮自动测试量程配置"(w811) -> ()
              }
              frame "总氮" {
                n477 = global write "总磷总氮断电保存全局变量.vi" "总氮自动测试量程配置"(w812) -> ()
              }
              frame "总磷" {
                n478 = global write "总磷总氮断电保存全局变量.vi" "总磷自动测试量程配置"(w813) -> ()
              }
            }
          }
          frame #1 {
            n479 = call "配置文件路径.vi"() -> ("appended path"=w814:path)  [unwired: 11 in]
            n480 = call <vilib>:"Open Config Data.vi"("configuration file path"=w814) -> ("error out"=w822:errorcluster, "refnum"=w825:T13)  [unwired: 8 in, 1 out]
            n481 = vi-ref "总磷总氮断电保存全局变量.vi"() -> (w824:refnum<vi>)
            n482 = call <userlib>:"Write Panel to INI__ogtk.vi"("error in (no error)"=w822, "VI ref"=w824, "refnum"=w825) -> ("error out"=w821:errorcluster, "refnum out"=w823:T13)  [unwired: 7 in]
            n483 = call <vilib>:"Close Config Data.vi"("error in (no error)"=w821, "refnum"=w823) -> ("error out"=w816:errorcluster, "file path"=w815:path)  [unwired: 8 in]
            n484 = Open/Create/Replace File(file path (use dialog)=w815, error in=w816) -> (refnum out=w819:refnum<file>, error out=w820:errorcluster)  [unwired: 4 in, 1 out]
            n485 = Flush File(refnum=w819, error in=w820) -> (refnum out=w818:refnum<file>, error out=w817:errorcluster)
            n486 = Close File(refnum=w818, error in=w817) -> ()  [unwired: 2 out]
          }
        }
      }
      event "手动启动": Value Change {
        n487 = event-data() -> ()  [unwired: 1 in, 6 out]
        n488 = call "总磷总氮启动参数对话框.vi"() -> ("确认"=w826:bool, "元素"=w827:cluster{"命令":string, "data":variant})  [unwired: 10 in]
        n489 = case shown="真" w826 {
          tunnel: w828 -> [_ w831]
          tunnel: w827 -> [_ w830]
          frame False {
          }
          frame True {
            n490 = Flush Queue(queue=w831) -> (queue out=w829:refnum<queue>)  [unwired: 1 in, 2 out]
            n491 = Enqueue Element(queue=w829, element=w830) -> ()  [unwired: 2 in, 3 out]
          }
        }
      }
      event "单步测试": Value Change {
        n492 = event-data() -> ()  [unwired: 1 in, 6 out]
        n493 = call "总磷单步调试对话框.vi"() -> ()  [unwired: 12 in]
      }
      event "停止": Value Change {
        n494 = event-data() -> ()  [unwired: 1 in, 6 out]
        n495 = Send Notification(notification=TRUE ("通知"), notifier=w833) -> ()  [unwired: 1 in, 2 out]
        n496 = Enqueue Element(queue=w837, element=cluster{"命令":string, "data":variant} {"命令"="启动", "data"=variant(cluster{"站号":u16, "控制命令输出":u16[]} {"站号"=1, "控制命令输出"=[2816]})} ("元素")) -> (queue out=w834:refnum<queue>)  [unwired: 2 in, 2 out]
        n497 = Enqueue Element(queue=w834, element=cluster{"命令":string, "data":variant} {"命令"="启动", "data"=variant(cluster{"站号":u16, "控制命令输出":u16[]} {"站号"=2, "控制命令输出"=[2816]})} ("元素")) -> ()  [unwired: 2 in, 3 out]
      }
      event "参数设置": Value Change {
        n498 = event-data() -> ()  [unwired: 1 in, 6 out]
        n499 = property on="窗格" class="Pane"("Origin"=T16 {"Horizontal"=0, "Vertical"=628} ("原点")) -> ()  [unwired: 2 in, 2 out]
      }
      event "返回": Value Change {
        n500 = event-data() -> ()  [unwired: 1 in, 6 out]
        n501 = property on="窗格" class="Pane"("Origin"=T16 {"Horizontal"=0, "Vertical"=0} ("原点")) -> ()  [unwired: 2 in, 2 out]
      }
      event "公式.X^2", "公式.X", "公式.b", "量程参数读取.测量精度", "量程参数读取.检出限", "量程参数读取.上限", "量程参数读取.下限", "量程参数读取.阈值（低->高）", "量程参数读取.阈值（高->低）", "量程参数读取.稀释度": Mouse Down {
        n502 = event-data() -> ("CtlRef"=w843:refnum<vi>)  [unwired: 1 in, 7 out]
        n503 = property class="DigNum (严格)"(reference=w843) -> (reference out=w841:refnum<vi>, "Value"=w842:dbl)  [unwired: 1 in, 1 out]
        n504 = call "数字键盘.vi"("OldNumber"=w842) -> ("NewNumber"=w840:dbl)
        n505 = property class="DigNum (严格)"(reference=w841, "Val(Sgnl)"=w840) -> ()  [unwired: 1 in, 2 out]
      }
      event "读公式": Value Change {
        n506 = event-data() -> ()  [unwired: 1 in, 6 out]
        n507 = property class="Enum (严格)"(reference=w851) -> ("Value"=w850:enum16{"COD", "氨氮", "总氮", "总磷"})  [unwired: 1 in, 2 out]
        n508 = property class="Enum (严格)"(reference=w852) -> ("Value"=w849:enum16{"水样测量", "零点核查", "跨度核查", "标样核查", "加标回收"})  [unwired: 1 in, 2 out]
        n509 = property class="Enum (严格)"(reference=w853) -> ("Value"=w848:enum16{"低量程", "高量程"})  [unwired: 1 in, 2 out]
        n510 = call "总磷总氮公式读取.vi"("量程"=w848, "测量模式"=w849, "测量参数"=w850) -> ("error out"=w845:errorcluster, "公式"=w846:cluster{"X^2":dbl, "X":dbl, "b":dbl})  [unwired: 7 in]
        n511 = property class="Clust (严格)"(reference=w847, "Value"=w846) -> ()  [unwired: 1 in, 2 out]
        n512 = case shown="错误" w845 {
          tunnel: ["读取成功" ("消息") "读取失败" ("消息")] -> w844
          frame No Error {
          }
          frame Error {
          }
        }
        n513 = One Button Dialog(message=w844) -> ()  [unwired: 1 in, 1 out]
      }
      event "写公式": Value Change {
        n514 = event-data() -> ()  [unwired: 1 in, 6 out]
        n515 = call "总磷总氮公式写入.vi"("公式"="公式", "量程"="量程下拉列表", "测量模式"="测量模式下拉列表", "测量参数"="参数下拉列表") -> ("error out"=w860:errorcluster)  [unwired: 7 in]
        n516 = case shown="无错误" w860 {
          tunnel: ["写入成功" ("消息") "写入失败" ("消息")] -> w861
          tunnel: "测量模式下拉列表" -> [w870 _]
          tunnel: "量程下拉列表" -> [w868 _]
          tunnel: "参数下拉列表" -> [w863 _]
          tunnel: "公式" -> [w862 _]
          frame No Error {
            n517 = Equal?(x=w870, y=enum16{"水样测量", "零点核查", "跨度核查", "标样核查", "加标回收"}."水样测量" ("测量模式下拉列表")) -> (x = y?=w866:bool)
            n518 = Equal?(x=w868, y=enum16{"低量程", "高量程"}."低量程" ("量程下拉列表")) -> (x = y?=w865:bool)
            n519 = And(x=w866, y=w865) -> (x .and. y?=w864:bool)
            n520 = case shown="真" w864 {
              tunnel: w863 -> [_ w873]
              tunnel: w862 -> [_ w872]
              frame False {
              }
              frame True {
                n521 = case shown="\"COD\"" w873 {
                  tunnel: w872 -> [w874 w880 w886 w892]
                  frame "总磷", Default {
                    n522 = Unbundle By Name(w874) -> ("X^2"=w877:dbl, "X"=w876:dbl, "b"=w875:dbl)
                    n523 = global read "总磷总氮断电保存全局变量.vi" "总磷仪器参数"() -> (w878:T27)
                    n524 = Bundle By Name(cluster=w878, "曲线截距"=w875, "曲线斜率"=w876, "二次多项式系数"=w877) -> (w879:T27)
                    n525 = global write "总磷总氮断电保存全局变量.vi" "总磷仪器参数"(w879) -> ()
                  }
                  frame "总氮" {
                    n526 = Unbundle By Name(w880) -> ("X^2"=w883:dbl, "X"=w882:dbl, "b"=w881:dbl)
                    n527 = global read "总磷总氮断电保存全局变量.vi" "总氮仪器参数"() -> (w884:T27)
                    n528 = Bundle By Name(cluster=w884, "曲线截距"=w881, "曲线斜率"=w882, "二次多项式系数"=w883) -> (w885:T27)
                    n529 = global write "总磷总氮断电保存全局变量.vi" "总氮仪器参数"(w885) -> ()
                  }
                  frame "COD" {
                    n530 = Unbundle By Name(w886) -> ("X^2"=w889:dbl, "X"=w888:dbl, "b"=w887:dbl)
                    n531 = global read "总磷总氮断电保存全局变量.vi" "COD仪器参数"() -> (w890:T27)
                    n532 = Bundle By Name(cluster=w890, "曲线截距"=w887, "曲线斜率"=w888, "二次多项式系数"=w889) -> (w891:T27)
                    n533 = global write "总磷总氮断电保存全局变量.vi" "COD仪器参数"(w891) -> ()
                  }
                  frame "氨氮" {
                    n534 = Unbundle By Name(w892) -> ("X^2"=w895:dbl, "X"=w894:dbl, "b"=w893:dbl)
                    n535 = global read "总磷总氮断电保存全局变量.vi" "氨氮仪器参数"() -> (w896:T27)
                    n536 = Bundle By Name(cluster=w896, "曲线截距"=w893, "曲线斜率"=w894, "二次多项式系数"=w895) -> (w897:T27)
                    n537 = global write "总磷总氮断电保存全局变量.vi" "氨氮仪器参数"(w897) -> ()
                  }
                }
              }
            }
          }
          frame Error {
          }
        }
        n538 = One Button Dialog(message=w861) -> ()  [unwired: 1 in, 1 out]
      }
      event "量程切换阈值读取": Value Change {
        n539 = event-data() -> ()  [unwired: 1 in, 6 out]
        n540 = property class="Enum (严格)"(reference=w904) -> ("Value"=w903:enum16{"COD", "氨氮", "总氮", "总磷"})  [unwired: 1 in, 2 out]
        n541 = call "总磷总氮量程读取.vi"("测量参数"=w903) -> ("error out"=w900:errorcluster, "量程参数读取"=w899:T29)  [unwired: 9 in]
        n542 = property class="Clust (严格)"(reference=w902, "Value"=w899) -> ()  [unwired: 1 in, 2 out]
        n543 = case shown="错误" w900 {
          tunnel: ["读取成功" ("消息") "读取失败" ("消息")] -> w901
          frame No Error {
          }
          frame Error {
          }
        }
        n544 = One Button Dialog(message=w901) -> ()  [unwired: 1 in, 1 out]
      }
      event "量程切换阈值写入": Value Change {
        n545 = event-data() -> ()  [unwired: 1 in, 6 out]
        n546 = property class="Enum (严格)"(reference=w911) -> ("Value"=w907:enum16{"COD", "氨氮", "总氮", "总磷"})  [unwired: 1 in, 2 out]
        n547 = call "总磷总氮量程写入.vi"("量程参数写入"="量程参数读取", "测量参数"=w907) -> ("error out"=w909:errorcluster)  [unwired: 8 in]
        n548 = case shown="无错误" w909 {
          tunnel: ["写入成功" ("消息") "写入失败" ("消息")] -> w910
          frame No Error {
          }
          frame Error {
          }
        }
        n549 = One Button Dialog(message=w910) -> ()  [unwired: 1 in, 1 out]
      }
    }
  }
